vi "main 0.9.3.testing.vi"() -> ()   [LabVIEW 2015]
uses:
  subvi/PHOIBOS/DEFINITIONS/DEF_dev_state.ctl
  subvi/PHOIBOS/DEFINITIONS/DEF_dev_type.ctl
  <vilib>/Analysis/1siggen.llb/Ramp Pattern by Samples.vi
  <vilib>/Utility/file.llb/Write Delimited Spreadsheet (DBL).vi
  <vilib>/Utility/file.llb/Read Delimited Spreadsheet (string).vi
  <vilib>/DAQmx/create/channels.llb/DAQmx Create Channel (AI-Voltage-Basic).vi
  subvi/Newport ESP301/Newport ESP301.lvlib
  subvi/sp_manip.llb/sp_manip_lib.lvlib
  subvi/sp_manip.llb/tcp_gateway.lvlib
  <vilib>/Analysis/NI_AALBase.lvlib
panel:
  in  "Frame trigger \n(High Performance and QE only)":u16
  in  "Operating mode\nHP & QE / HS & DiCam Pro":u32
  out "Waveform Chart":dbl(graph)
  out "G2 X":cluster{dbl[], "Ramp Pattern":dbl[]}(graph)={array[344 elements], "Ramp Pattern"=[5593.0, 5541.0, 5578.0, 5573.0, 5542.0, 5582.0, 5523.0, 5570.0, 5578.0, 5560.0, 5581.0, 5542.0, 5577.0, 5517.0, 5599.0, 5558.0, 5549.0, 5571.0, 5527.0, 5574.0, 5565.0, 5561.0, 5570.0, 5531.0, 5576.0, 5531.0, 5576.0, 5554.0, 5523.0, 5573.0, 5536.0, 5555.0, 5539.0, 5549.0, 5543.0, 5541.0, 5581.0, 5523.0, 5548.0, 5528.0, 5558.0, 5565.0, 5537.0, 5556.0, 5521.0, 5538.0, 5549.0, 5532.0, 5562.0, 5512.0, 5555.0, 5549.0, 5536.0, 5542.0, 5511.0, 5567.0, 5526.0, 5549.0, 5545.0, 5543.0, 5562.0, 5518.0, 5561.0, 5490.0, 5542.0, 5522.0, 5529.0, 5542.0, 5521.0, 5556.0, 5511.0, 5541.0, 5534.0, 5512.0, 5569.0, 5525.0, 5547.0, 5507.0, 5533.0, 5533.0, 5501.0, 5555.0, 5497.0, 5517.0, 5526.0, 5519.0, 5565.0, 5503.0, 5548.0, 5496.0, 5544.0, 5523.0, 5534.0, 5533.0, 5501.0, 5529.0, 5494.0, 5523.0, 5526.0, 5519.0, 5539.0, 5493.0, 5508.0, 5532.0, 5504.0, 5546.0, 5540.0, 5550.0, 5488.0, 5556.0, 5535.0, 5510.0, 5535.0, 5515.0, 5543.0, 5475.0, 5538.0, 5528.0, 5504.0, 5523.0, 5502.0, 5535.0, 5473.0, 5503.0, 5501.0, 5531.0, 5525.0, 5490.0, 5524.0, 5484.0, 5520.0, 5506.0, 5492.0, 5516.0, 5477.0, 5511.0, 5487.0, 5509.0, 5496.0, 5467.0, 5538.0, 5494.0, 5512.0, 5497.0, 5498.0, 5526.0, 5482.0, 5506.0, 5466.0, 5522.0, 5489.0, 5512.0, 5518.0, 5475.0, 5547.0, 5480.0, 5569.0, 5504.0, 5485.0, 5528.0, 5506.0, 5529.0, 5468.0, 5524.0, 5507.0, 5518.0, 5511.0, 5471.0, 5525.0, 5480.0, 5482.0, 5510.0, 5506.0, 5522.0, 5475.0, 5540.0, 5477.0, 5511.0, 5514.0, 5500.0, 5497.0, 5484.0, 5536.0, 5476.0, 5485.0, 5527.0, 5509.0, 5529.0, 5495.0, 5504.0, 5496.0, 5519.0, 5512.0, 5469.0, 5506.0, 5465.0, 5502.0, 5481.0, 5508.0, 5519.0, 5499.0, 5515.0, 5476.0, 5496.0, 5502.0, 5499.0, 5494.0, 5477.0, 5541.0, 5477.0, 5512.0, 5497.0, 5472.0, 5511.0, 5471.0, 5503.0, 5507.0, 5504.0, 5477.0, 5479.0, 5508.0, 5481.0, 5522.0, 5517.0, 5516.0, 5505.0, 5502.0, 5491.0, 5481.0, 5512.0, 5484.0, 5500.0, 5478.0, 5493.0, 5529.0, 5492.0, 5518.0, 5471.0, 5518.0, 5490.0, 5513.0, 5497.0, 5488.0, 5517.0, 5477.0, 5524.0, 5464.0, 5495.0, 5514.0, 5495.0, 5522.0, 5477.0, 5490.0, 5535.0, 5489.0, 5491.0, 5491.0, 5515.0, 5473.0, 5504.0, 5505.0, 5515.0, 5510.0, 5473.0, 5521.0, 5475.0, 5537.0, 5499.0, 5505.0, 5509.0, 5460.0, 5509.0, 5473.0, 5489.0, 5500.0, 5464.0, 5522.0, 5471.0, 5528.0, 5475.0, 5502.0, 5494.0, 5511.0, 5516.0, 5486.0, 5528.0, 5471.0, 5492.0, 5477.0, 5491.0, 5531.0, 5486.0, 5549.0, 5498.0, 5524.0, 5482.0, 5495.0, 5505.0, 5476.0, 5512.0, 5444.0, 5512.0, 5498.0, 5471.0, 5489.0, 5462.0, 5502.0, 5459.0, 5503.0, 5489.0, 5493.0, 5498.0, 5461.0, 5505.0, 5495.0, 5503.0, 5459.0, 5501.0, 5515.0, 5459.0, 5510.0, 5469.0, 5504.0, 5499.0, 5505.0, 5524.0, 5477.0, 5527.0, 5477.0, 5475.0, 5495.0, 5482.0, 5514.0, 5481.0, 5499.0, 5481.0, 5482.0, 5498.0, 5460.0, 5469.0, 5471.0, 5519.0, 5495.0, 5485.0]}
  in  "reset every n pics":bool
  in  "pics2avg":i32=50
  in  "abort acq.":bool
  out "G2 Y":cluster{dbl[], "Ramp Pattern":dbl[]}(graph)={[5738.0, 5692.0, 5562.0, 5630.0, 5633.0, 5616.0, 5523.0, 5622.0, 5406.0, 5598.0, 5416.0, 5403.0, 5579.0, 5325.0, 5504.0, 5402.0, 5538.0, 5568.0, 5460.0, 5494.0, 5367.0, 5597.0, 5434.0, 5448.0, 5339.0, 5434.0, 5460.0, 5482.0, 5646.0, 5720.0, 5704.0, 5628.0, 5672.0, 5511.0, 5420.0, 5539.0, 5543.0, 5421.0, 5486.0, 5508.0, 5537.0, 5586.0, 5460.0, 5547.0, 5433.0, 5488.0, 5552.0, 5538.0, 5528.0, 5482.0, 5406.0, 5458.0, 5644.0, 5485.0, 5443.0, 5485.0, 5385.0, 5413.0, 5472.0, 5571.0, 5640.0, 5602.0, 5462.0, 5477.0, 5408.0, 5396.0, 5445.0, 5638.0, 5383.0, 5571.0, 5372.0, 5519.0, 5426.0, 5462.0, 5481.0, 5626.0, 5326.0, 5458.0, 5471.0, 5366.0, 5394.0, 5363.0, 5551.0, 5596.0, 5452.0, 5470.0, 5600.0, 5533.0, 5573.0, 5544.0, 5671.0, 5595.0, 5423.0, 5550.0, 5557.0, 5416.0, 5404.0, 5478.0, 5448.0, 5512.0, 5505.0, 5575.0, 5434.0, 5436.0, 5600.0, 5487.0, 5607.0, 5463.0, 5606.0, 5540.0, 5521.0, 5581.0, 5472.0, 5555.0, 5576.0, 5612.0, 5529.0, 5473.0, 5454.0, 5455.0, 5500.0, 5650.0, 5451.0, 5445.0, 5423.0, 5376.0, 5389.0, 5491.0, 5536.0, 5525.0, 5440.0, 5707.0, 5414.0, 5532.0, 5400.0, 5668.0, 5706.0, 5515.0, 5431.0, 5400.0, 5439.0, 5471.0, 5627.0, 5691.0, 5569.0, 5718.0, 5614.0, 5523.0, 5436.0, 5432.0, 5419.0, 5516.0, 5469.0, 5467.0, 5530.0, 5598.0, 5501.0, 5476.0, 5457.0, 5460.0, 5606.0, 5456.0, 5429.0, 5586.0, 5504.0, 5546.0, 5516.0, 5466.0, 5650.0, 5593.0, 5605.0, 5515.0, 5414.0, 5623.0, 5581.0, 5651.0, 5574.0, 5519.0, 5672.0, 5621.0, 5496.0, 5382.0, 5496.0, 5620.0, 5542.0, 5422.0, 5492.0, 5515.0, 5549.0, 5402.0, 5472.0, 5547.0, 5515.0, 5641.0, 5451.0, 5667.0, 5622.0, 5511.0, 5506.0, 5608.0, 5647.0, 5584.0, 5714.0, 5490.0, 5534.0, 5463.0, 5566.0, 5573.0, 5570.0, 5582.0, 5613.0, 5504.0, 5550.0, 5594.0, 5576.0, 5677.0, 5675.0, 5681.0, 5681.0, 5434.0, 5434.0, 5405.0, 5473.0, 5522.0, 5427.0, 5533.0, 5582.0, 5427.0, 5529.0, 5548.0, 5341.0, 5521.0, 5539.0, 5435.0, 5457.0, 5511.0, 5406.0, 5412.0, 5620.0, 5609.0, 5609.0, 5469.0, 5577.0, 5661.0, 5673.0, 5518.0, 5463.0, 5562.0, 5723.0, 5719.0, 5487.0, 5485.0, 5683.0, 5501.0, 5604.0, 5328.0], "Ramp Pattern"=[0.0, 1.003921568627451, 2.007843137254902, 3.011764705882353, 4.015686274509804, 5.019607843137255, 6.023529411764706, 7.027450980392157, 8.031372549019608, 9.035294117647059, 10.03921568627451, 11.04313725490196, 12.047058823529412, 13.050980392156863, 14.054901960784314, 15.058823529411764, 16.062745098039215, 17.066666666666666, 18.070588235294117, 19.07450980392157, 20.07843137254902, 21.08235294117647, 22.08627450980392, 23.090196078431372, 24.094117647058823, 25.098039215686274, 26.101960784313725, 27.105882352941176, 28.109803921568627, 29.113725490196078, 30.11764705882353, 31.12156862745098, 32.12549019607843, 33.129411764705885, 34.13333333333333, 35.13725490196079, 36.141176470588235, 37.14509803921569, 38.14901960784314, 39.15294117647059, 40.15686274509804, 41.16078431372549, 42.16470588235294, 43.168627450980395, 44.17254901960784, 45.1764705882353, 46.180392156862744, 47.1843137254902, 48.188235294117646, 49.1921568627451, 50.19607843137255, 51.2, 52.20392156862745, 53.207843137254905, 54.21176470588235, 55.21568627450981, 56.219607843137254, 57.22352941176471, 58.227450980392156, 59.23137254901961, 60.23529411764706, 61.23921568627451, 62.24313725490196, 63.247058823529414, 64.25098039215686, 65.25490196078431, 66.25882352941177, 67.26274509803922, 68.26666666666667, 69.27058823529411, 70.27450980392157, 71.27843137254902, 72.28235294117647, 73.28627450980392, 74.29019607843138, 75.29411764705883, 76.29803921568627, 77.30196078431372, 78.30588235294118, 79.30980392156863, 80.31372549019608, 81.31764705882352, 82.32156862745099, 83.32549019607843, 84.32941176470588, 85.33333333333333, 86.33725490196079, 87.34117647058824, 88.34509803921569, 89.34901960784313, 90.3529411764706, 91.35686274509804, 92.36078431372549, 93.36470588235294, 94.3686274509804, 95.37254901960785, 96.37647058823529, 97.38039215686274, 98.3843137254902, 99.38823529411765, 100.3921568627451, 101.39607843137254, 102.4, 103.40392156862745, 104.4078431372549, 105.41176470588235, 106.41568627450981, 107.41960784313726, 108.4235294117647, 109.42745098039215, 110.43137254901961, 111.43529411764706, 112.43921568627451, 113.44313725490196, 114.44705882352942, 115.45098039215686, 116.45490196078431, 117.45882352941176, 118.46274509803922, 119.46666666666667, 120.47058823529412, 121.47450980392156, 122.47843137254903, 123.48235294117647, 124.48627450980392, 125.49019607843137, 126.49411764705883, 127.49803921568628, 128.50196078431372, 129.50588235294117, 130.50980392156862, 131.51372549019607, 132.51764705882354, 133.521568627451, 134.52549019607844, 135.52941176470588, 136.53333333333333, 137.53725490196078, 138.54117647058823, 139.54509803921567, 140.54901960784315, 141.5529411764706, 142.55686274509804, 143.5607843137255, 144.56470588235294, 145.5686274509804, 146.57254901960783, 147.57647058823528, 148.58039215686276, 149.5843137254902, 150.58823529411765, 151.5921568627451, 152.59607843137255, 153.6, 154.60392156862744, 155.6078431372549, 156.61176470588236, 157.6156862745098, 158.61960784313726, 159.6235294117647, 160.62745098039215, 161.6313725490196, 162.63529411764705, 163.6392156862745, 164.64313725490197, 165.64705882352942, 166.65098039215687, 167.65490196078431, 168.65882352941176, 169.6627450980392, 170.66666666666666, 171.6705882352941, 172.67450980392158, 173.67843137254903, 174.68235294117648, 175.68627450980392, 176.69019607843137, 177.69411764705882, 178.69803921568626, 179.7019607843137, 180.7058823529412, 181.70980392156864, 182.71372549019608, 183.71764705882353, 184.72156862745098, 185.72549019607843, 186.72941176470587, 187.73333333333332, 188.7372549019608, 189.74117647058824, 190.7450980392157, 191.74901960784314, 192.75294117647059, 193.75686274509803, 194.76078431372548, 195.76470588235293, 196.7686274509804, 197.77254901960785, 198.7764705882353, 199.78039215686275, 200.7843137254902, 201.78823529411764, 202.7921568627451, 203.79607843137254, 204.8, 205.80392156862746, 206.8078431372549, 207.81176470588235, 208.8156862745098, 209.81960784313725, 210.8235294117647, 211.82745098039214, 212.83137254901962, 213.83529411764707, 214.8392156862745, 215.84313725490196, 216.8470588235294, 217.85098039215686, 218.8549019607843, 219.85882352941175, 220.86274509803923, 221.86666666666667, 222.87058823529412, 223.87450980392157, 224.87843137254902, 225.88235294117646, 226.8862745098039, 227.89019607843136, 228.89411764705883, 229.89803921568628, 230.90196078431373, 231.90588235294118, 232.90980392156862, 233.91372549019607, 234.91764705882352, 235.92156862745097, 236.92549019607844, 237.9294117647059, 238.93333333333334, 239.93725490196078, 240.94117647058823, 241.94509803921568, 242.94901960784313, 243.95294117647057, 244.95686274509805, 245.9607843137255, 246.96470588235294, 247.9686274509804, 248.97254901960784, 249.9764705882353, 250.98039215686273, 251.98431372549018, 252.98823529411766, 253.9921568627451, 254.99607843137255, 256.0]}
  out "ETA":timestamp=timestamp(3543843884.995538 s since 1904-01-01) format="%<%H:%M:%S>T"
  out "acq. imgs":i32=30
  out "snap_prog":dbl(slide)=1.0 scale=0.0..1.0
  in  "BasePath":path=path "Z:/PESdata"
  in  "cam_liveavg":bool caption="live average"
  out "cam_fps":dbl=20.079713544692744 caption="FPS" format="%.1g"
  out "sideimg":dbl[][](graph)
  in  "RunNumber":u16=77
  out "sum":dbl=4126991.0 format="%#.2g"
  out "max":dbl=54.0
  out "mainimg":dbl[][](graph)
  out "ESP_con?":bool=TRUE caption="ESP301"
  out "phoib_con?":bool caption="PHOIBOS"
  out "manip_con?":bool caption="manipulator"
  out "cam_con?":bool caption="camera"
  in  "main_close":bool
  in  "Tab Control":T1(tab)
  in  "manip_deltas":dbl[](array[numeric])=[0.0, 0.0, 0.0, 0.0, 10.0, 0.0] caption="delta" format="%#.5g"
  in  "aq.mode":enum32{"Radio Selection 1", "Radio Selection 2"}(radio)=enum."Radio Selection 2"
  in  "dark avg":i32=100
  in  "averages":i32=30 caption="N"
  in  "ESP_delta":dbl caption="relative [mm]"
  in  "ESP_-":bool
  in  "ESP_+":bool
  in  "ESP_go":bool
  in  "ESP_dest_t":dbl=250.17307139859977 caption="[fs]"
  in  "ESP_dest":dbl=31.304 caption="[mm]"
  in  "ESP_set_t0":bool
  in  "phoib_I_6s":dbl=3200.0
  in  "phoib_I_5s":dbl=1650.0
  in  "phoib_I_4s":dbl=4.558
  in  "phoib_I_3s":dbl=-7.0
  in  "phoib_I_2s":dbl=20.0
  in  "phoib_I_1s":dbl=22.0
  in  "phoib_standby":bool
  in  "phoib_set":bool
  out "phoib_I_6":dbl caption="Screen Voltage"
  out "phoib_I_5":dbl caption="Detctor Voltage"
  out "phoib_I_4":dbl caption="Work Function"
  out "phoib_I_3":dbl caption="Coil Current"
  out "phoib_I_2":dbl caption="Pass Energy"
  out "phoib_I_1":dbl caption="Kinetic Energy"
  out "Saved Positions":string[][](table)=[["ertwertwert", "-2.299945", "-2.030214", "38.900024", "50.000762", "0.000887", "-97.998082"], ["uztgugt", "-14.999451", "-13.638894", "442.380066", "13.998380", "-1.893758", "-76.305838"], ["asdf", "-14.999451", "-13.638894", "442.380066", "13.998380", "-1.893758", "-76.305838"], ["test3", "-14.999451", "-13.638894", "441.380066", "13.998380", "-1.893758", "-76.305838"]]
  in  "Save Pos":bool
  in  "Load":bool
  in  "Delete":bool
  in  "ManipRel +":bool
  in  "ManipRel -":bool
  in  "Move Abs":bool
  in  "stop manip":bool
  in  "dest":dbl[](array[numeric])=[-2.6172862113166087, -0.009888298846365134, 68.5008544921875, -46.36280498847848, 1.1073518432055398, -218.56360350415366] caption="destination" format="%#.5g"
  out "axis":string[](array[string])=["x", "y", "z", "polar", "tilt", "azimut"]
  out "pos":dbl[](array[numeric])=[-2.6172862113166087, -0.009888298846365134, 68.5008544921875, -46.363686276590336, 11.108982061941884, -218.56360350415366] caption="position" format="%.5f"
  in  "Mode":T2(ring)=enum."WideAngleMode"
  in  "VoltageRange":enum16{"3.5kV", "1.5kV", "400V", "100V", "10V"}(ring)=enum."400V"
  out "ESP_pos":dbl=31.4539 caption="Position"
  out "ESP_delay":dbl=1000.0251574040756 caption="Delay"
  out "ESP_t0":dbl=31.304 caption="Time Zero @"
  out "phoib_I_7":dbl caption="Conversion Voltage"
  in  "phoib_I_7s":dbl=-16.0
  in  "phoib_I_8s":dbl=0.0039
  in  "phoib_I_9s":dbl=0.0039
  out "phoib_I_8":dbl caption="FD1"
  out "phoib_I_9":dbl caption="FD2"
  in  "gain":bool
  in  "exposure [ms]":u32=1
  in  "binning":u16(ring)=2 items=["X 1", "X 2", "X 4", "X 8"]
  in  "cam_dark?":bool caption="subtract dark?"
  in  "cam_dark":bool
  in  "cam_saveimg":bool
  in  "e-size":u8
  in  "lower threshold":i32=-100
  in  "count?":bool
  in  "ROI Left":i32=1
  in  "ROI Right":i32=43
  in  "ROI Top":i32=1
  in  "ROI Bottom":i32=33
  out "moving?":bool[](array[boolean])
  in  "delscan_abort 2":bool
  in  "delscan_go 2":bool
  in  "delscan_finishIteration 2":bool
  out "del_ETA":timestamp=timestamp(3543843871.185777 s since 1904-01-01) format="%<%H:%M:%S>T"
  out "time / step":dbl=2.792118032773336
  out "duration [HH:MM:SS]":dbl=55.62603882380894 format="%<%H:%M:%S>t"
  out "disk [MB]":dbl=11.613000000000001
  out "RAM [MB]":dbl=2.765
  out "total steps":dbl=20.0
  out "delaypoints":dbl=5.0
  in  "generate delay table":bool
  in  "load delay table":bool
  in  "delay table [fs]":string[][](table)=[["-1000.000000"], ["-500.000000"], ["0.000000"], ["500.000000"], ["1000.000000"]]
  in  "delscan_iters":u32=4 caption="iterations"
  out "scangraph":cluster{"delaypoints":dbl[], dbl[]}(graph)={"delaypoints"=[-1000.0, -500.0, 0.0, 500.0, 1000.0], [56872639.0, 56944859.59999999, 56835838.7999999, 56879783.599999934, 56864774.39999998]}
  in  "delscan_abort":bool
  out "delscan_progress":u32(slide)=5 scale=0.0..5.0
  in  "delscan_go":bool
  out "delscan_pos":dbl=31.453896228999998 caption="stage pos [mm]"
  in  "delscan_end":dbl=1000.0 caption="end [fs]"
  in  "delscan_stepsize":dbl=500.0 caption="stepsize [fs]"
  in  "delscan_start":dbl=-1000.0 caption="start [fs]"
  out "iteration":i32=5
  in  "delscan_finishIteration":bool
  in  "manip_scan_steps":u32=3
  in  "Optimize":bool
  in  "manip_scan_delta":dbl[](array[numeric])=[0.0, 0.0, 0.0, 0.0, 1.0, 0.0] caption="delta" format="%#.5g"
  out "delscan_progress 2":u32(slide)=2 scale=0.0..3.0
  in  "abort":bool
  in  "dev_bench":bool
  out "x/y":dbl
  out "1/x":dbl
  in  "stop":bool
  out "voltage out":dbl
  out "sideimg 2":i32[][](graph)
  in  "manip_init":bool
  in  "manip_release":bool
  in  "phoib_init":bool
  in  "phoib_release":bool
  in  "ESP_init":bool
  in  "ESP_release":bool
  in  "ESP301 VISA":refnum<visa-resource-name>="COM8"
  in  "board number":i32
  in  "cam_init":bool
  in  "cam_release":bool
  out "cam_error":errorcluster
  out "phoib_error":errorcluster
  out "state":T3 items=["Off"=-1, "Standby"=0, "On"=1]
  in  "ESP Axis":i32=1 min=1 max=3
  out "error out":errorcluster
  out "error out 2":errorcluster={"status"=TRUE, "code"=1, "source"="TCP Write in sp_manip_lib.lvlib:sp_manip_disconnect.vi->main 0.9.1.vi"}
  # "0 = sequential\n1 = simultaneous"
  # "0 = internal\n1 = external rising\n2 = external falling"
  # "camera"
  # "analyzer"
  # "manipulator"
  # "aquisition"
  # "delay stage"
  # "Position"
  # "Destination"
  # "X\nY\nZ\npolar\ntilt\nazimut"
  # "camera"
  # "phoibos"
  # "ESP301"
  # "manipulator"
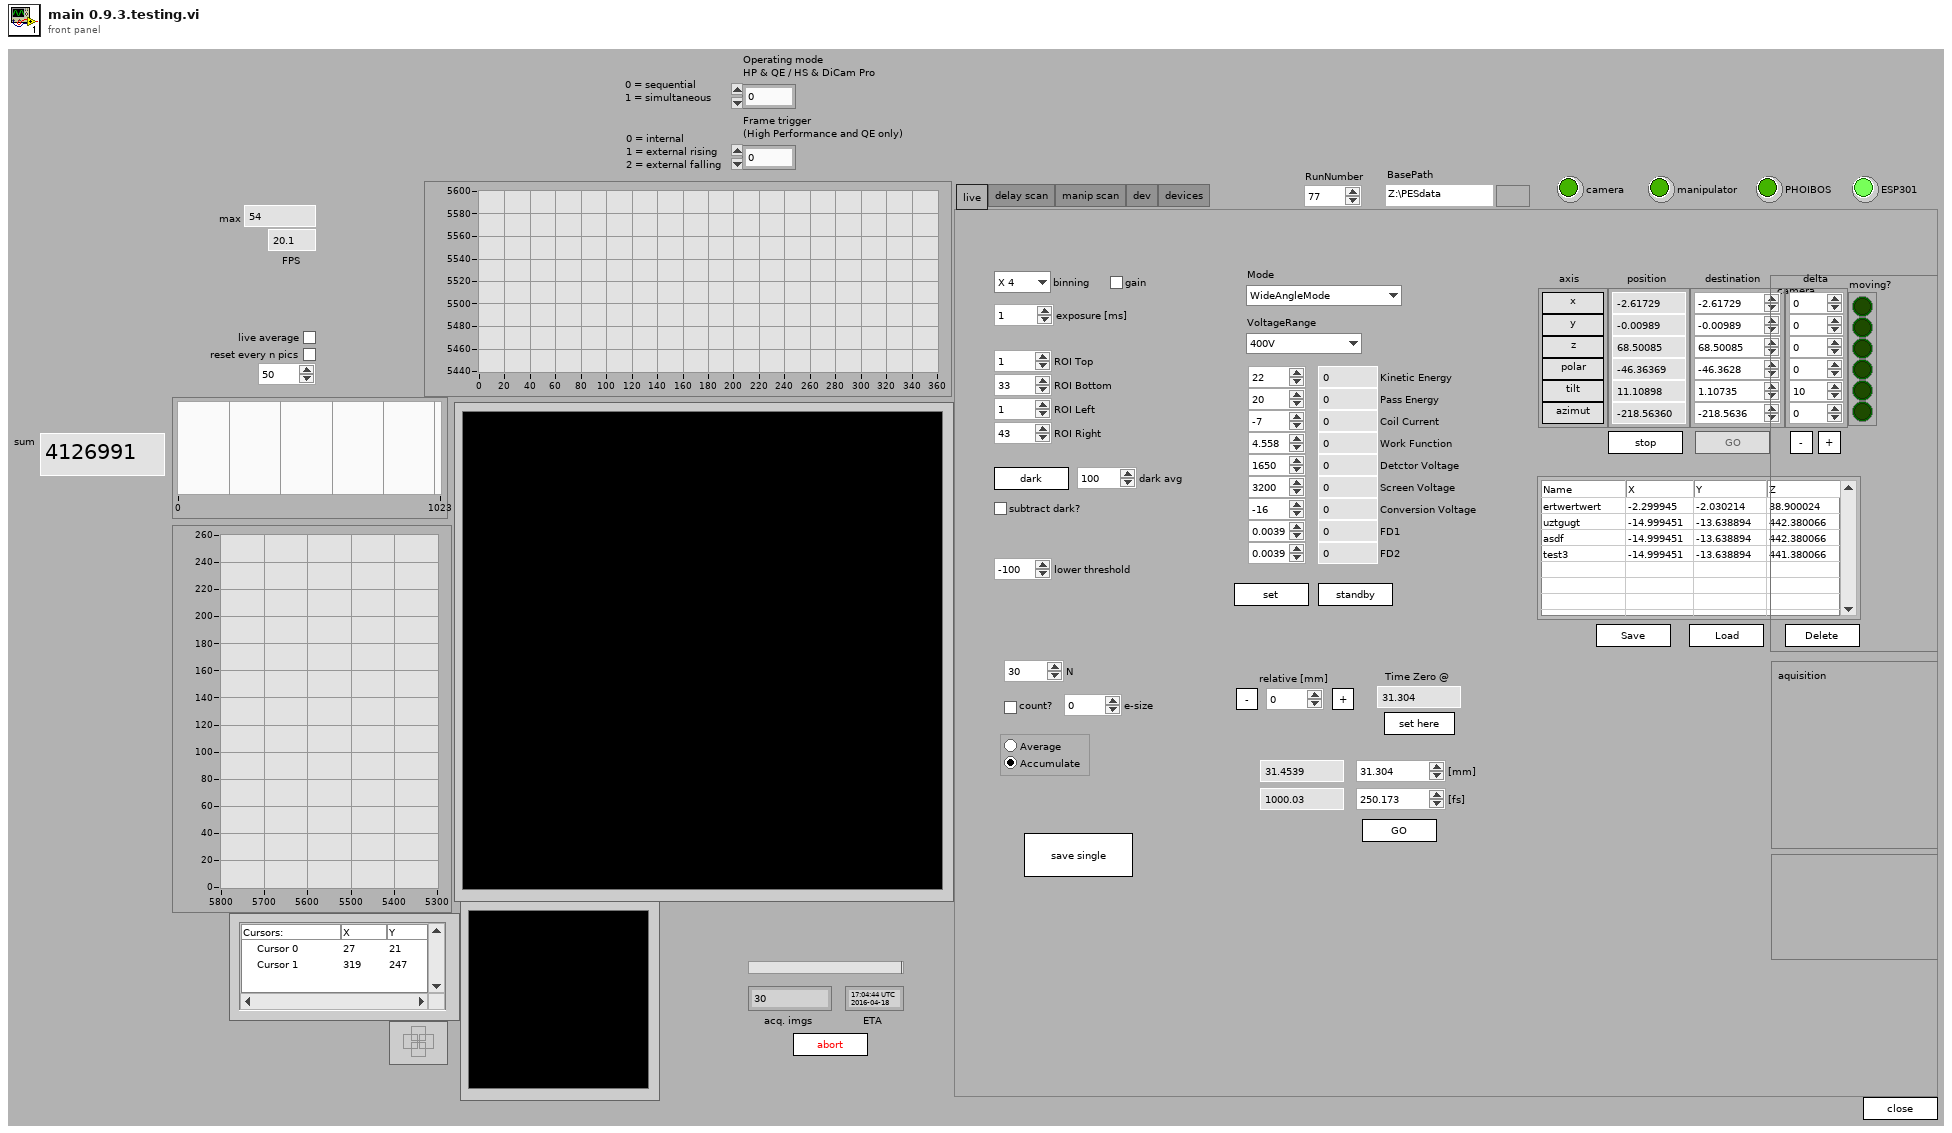
[diagram p1: front panel]
types:
  T1 = enum32{"live", "delay scan", "manip scan", "dev", "devices"}
  T2 = enum16{"HighMagnification", "MediumMagnification", "LowMagnification", "HighAngularDispersion", "MediumAngularDispersion", "LowAngularDispersion", "WideAngleMode", "LargeArea", "MediumArea", "SmallArea", "HighMagnification2", "SmallArea2", "ImagingMode"}
  T3 = typedef "DEF_dev_state.ctl" = i32
  T4 = typedef "LVCursorListTypeDef.ctl" = cluster{"Name":string, "Color":u32, "Style":u8, "Point Style":u8, "Name Visible":bool, "Allow Drag":bool, "Cursor Mode":u32, "Plot":i32, "Index":i32, "Position":cluster{"X":dbl, "Y":dbl}, "X Scale":u32, "Y Scale":u32, "Watch Plots":i32[], "Watch All Plots":bool, "Plot Area":i32, "Label Offset":cluster{"X":dbl, "Y":dbl}}[]
  T5 = cluster{"delay pointss [fs]":dbl[], "Intensity Chart":dbl[]}
  T6 = cluster{"Camera type":u32, "Operating mode\nHP & QE / HS & DiCam Pro ":u32, "Frame trigger \n(High Performance and QE only)":u16, "Sequence trigger":u16, "Low Light\n(QE only)":bool, "Gain":bool, "Horzontal\nbinning":u16, "Vertical\nbinning ":u16, "ROI Left":i32, "ROI Right":i32, "ROI Top":i32, "ROI Bottom":i32}
  T7 = cluster{"Name":string, "Color":u32, "Style":u8, "Point Style":u8, "Name Visible":bool, "Allow Drag":bool, "Cursor Mode":u32, "Plot":i32, "Index":i32, "Position":cluster{"X":dbl, "Y":dbl}, "X Scale":u32, "Y Scale":u32, "Watch Plots":i32[], "Watch All Plots":bool, "Plot Area":i32, "Label Offset":cluster{"X":dbl, "Y":dbl}}
  T8 = cluster{"Axis_Name":string, "Axis_Type":string, "Axis_Position":dbl, "continous":bool, "moving":bool}[]
  T9 = typedef "DEF_dev_type.ctl" = enum32{"devA (analyzer)", "devD (detector)"}
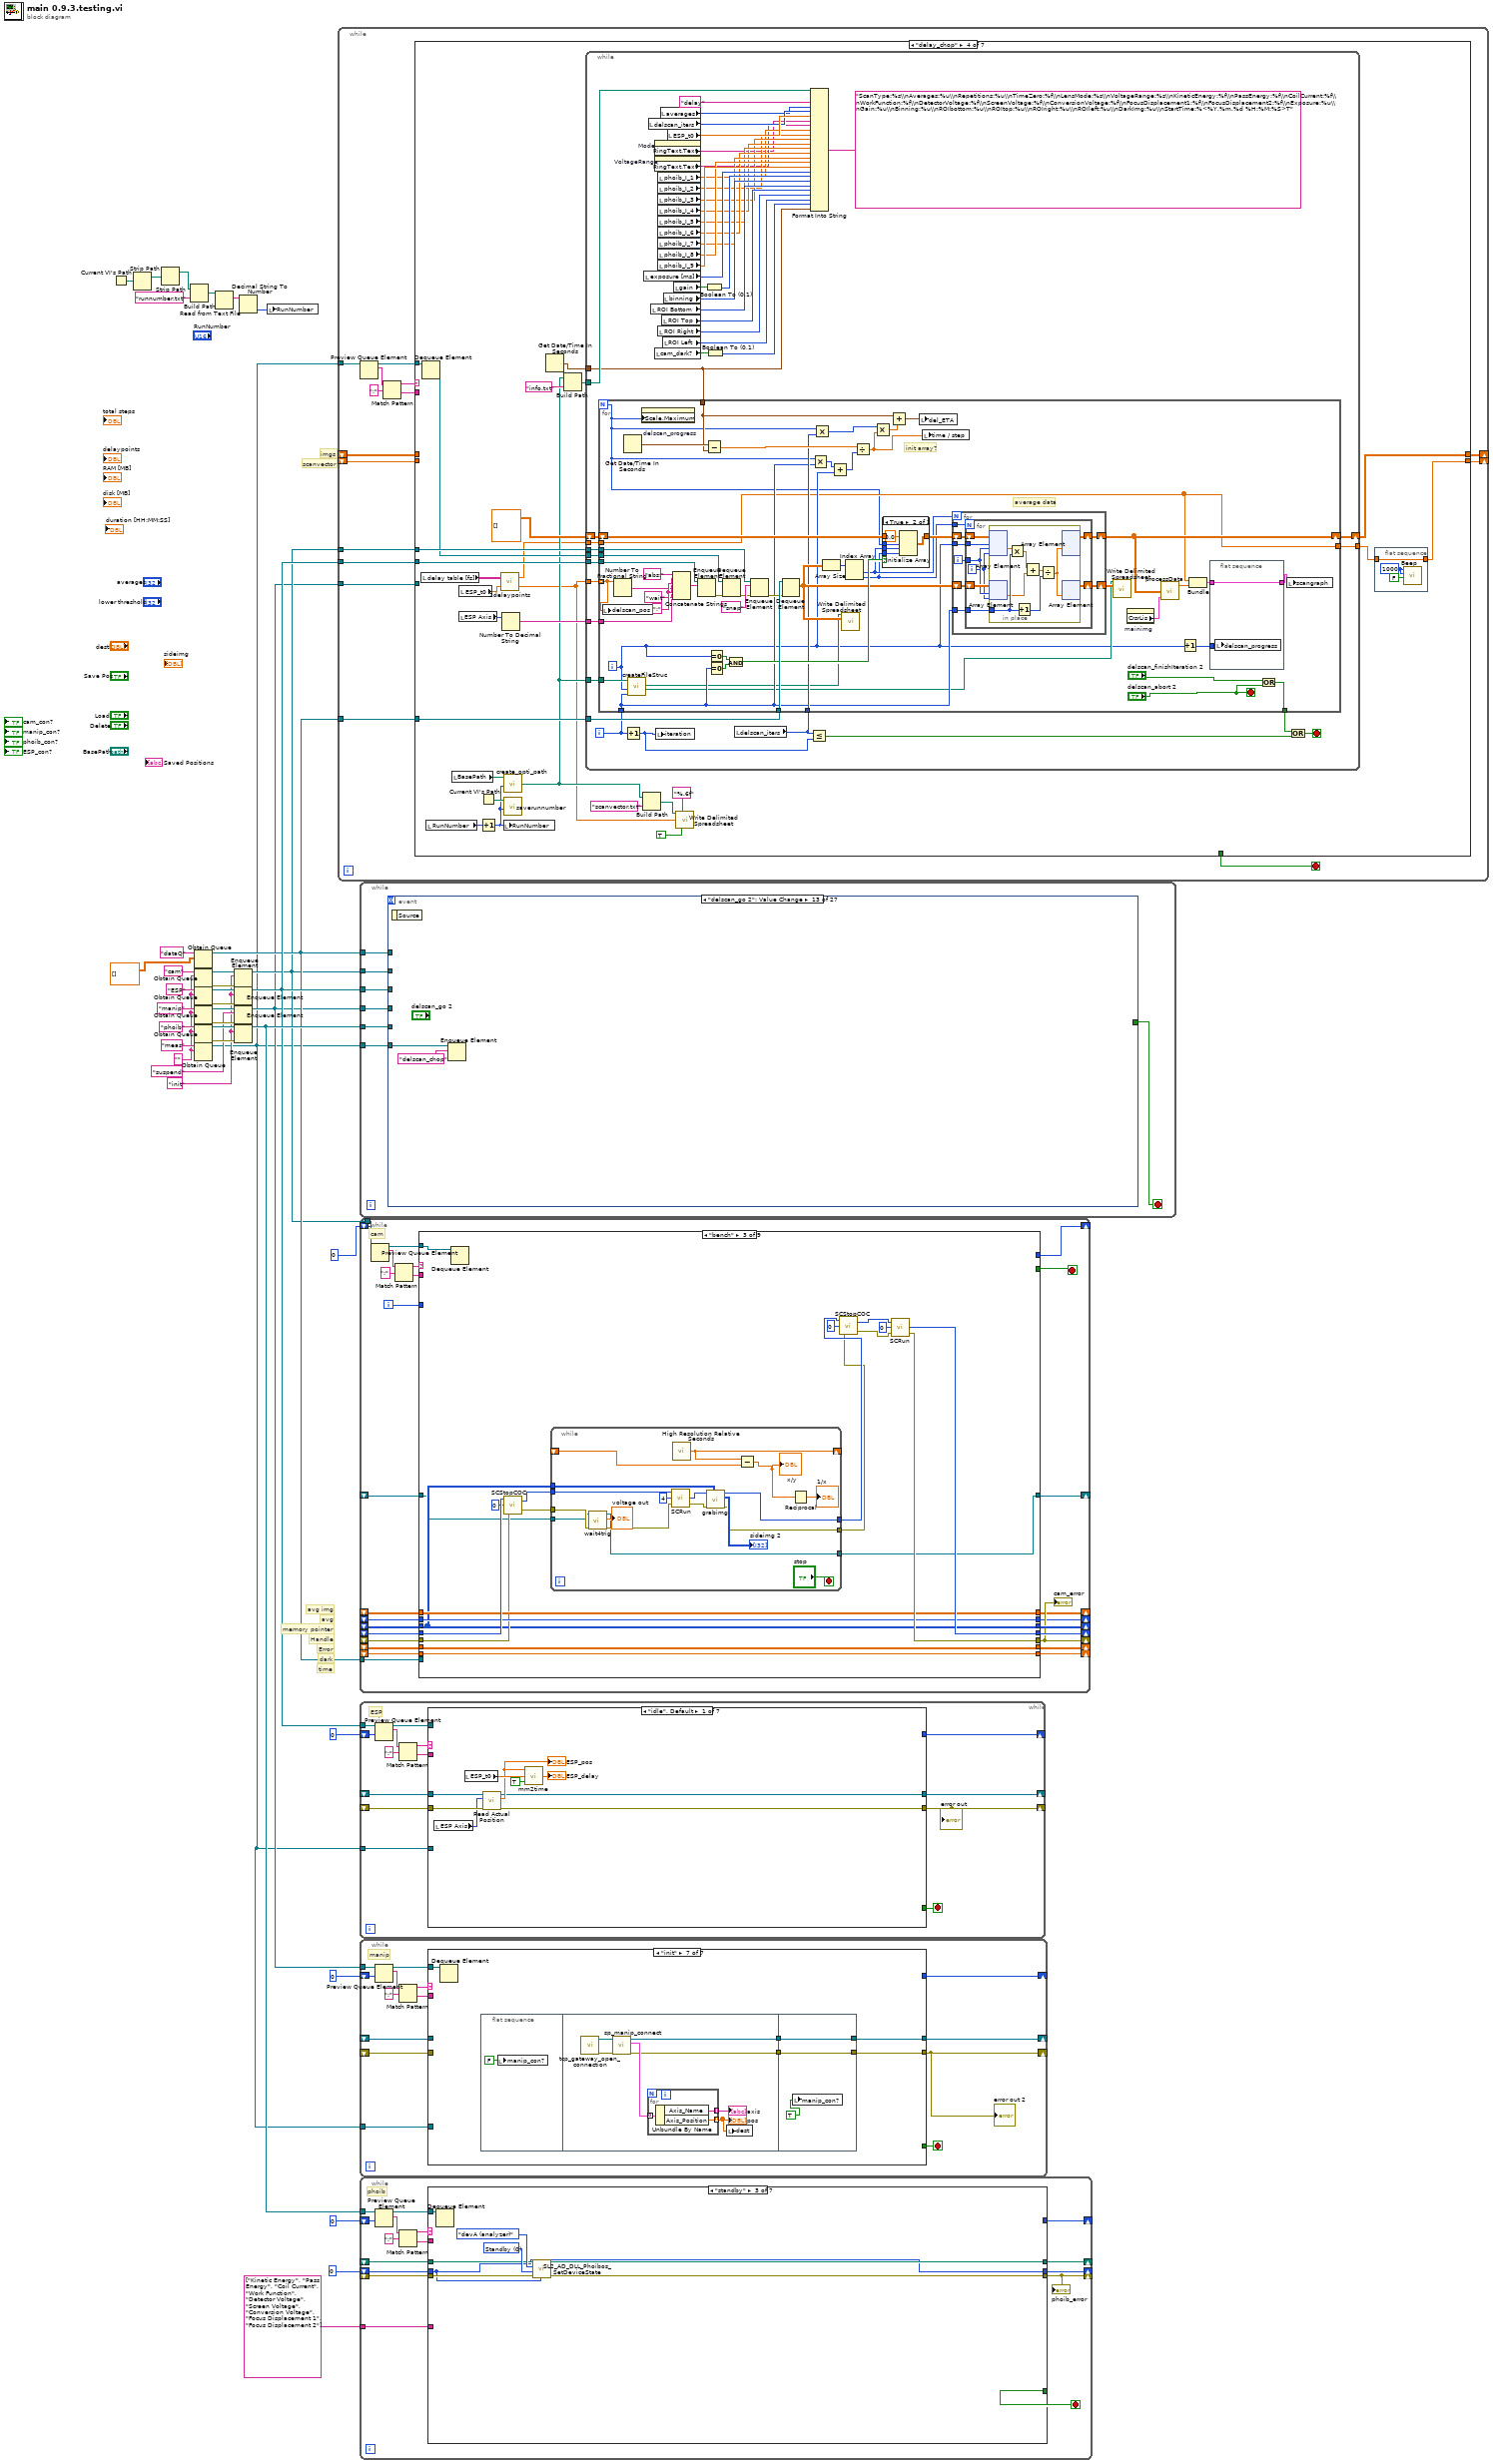
[diagram p0: block diagram]
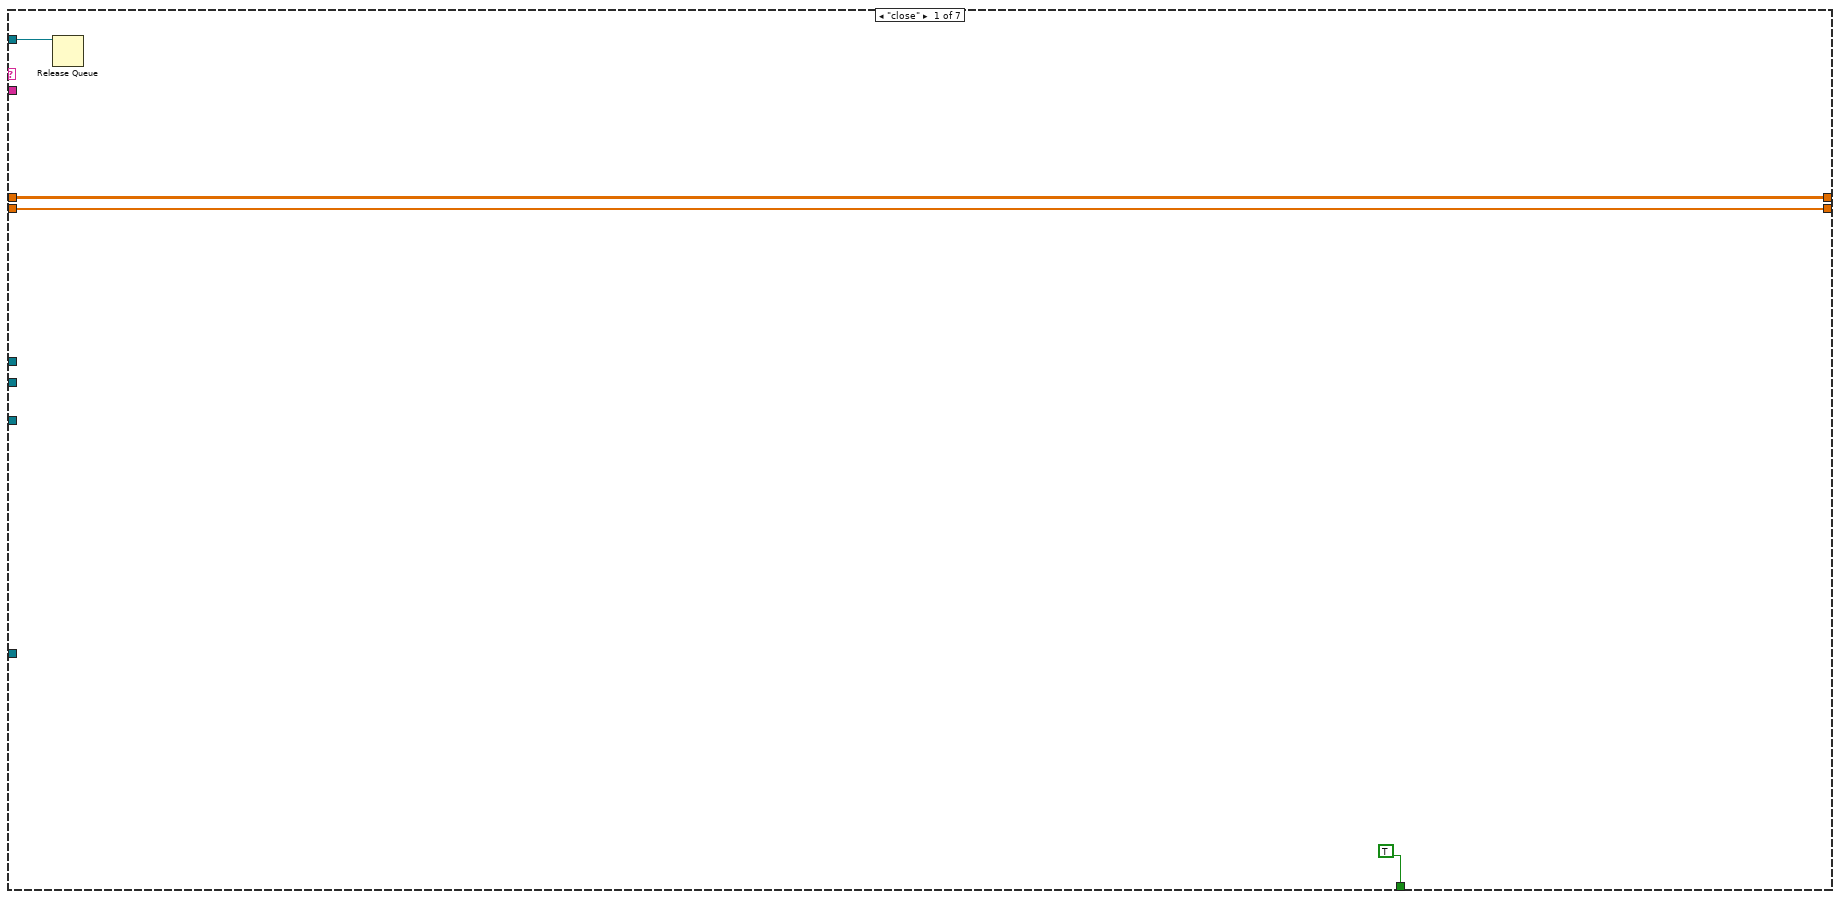
[diagram p2: hidden frame]
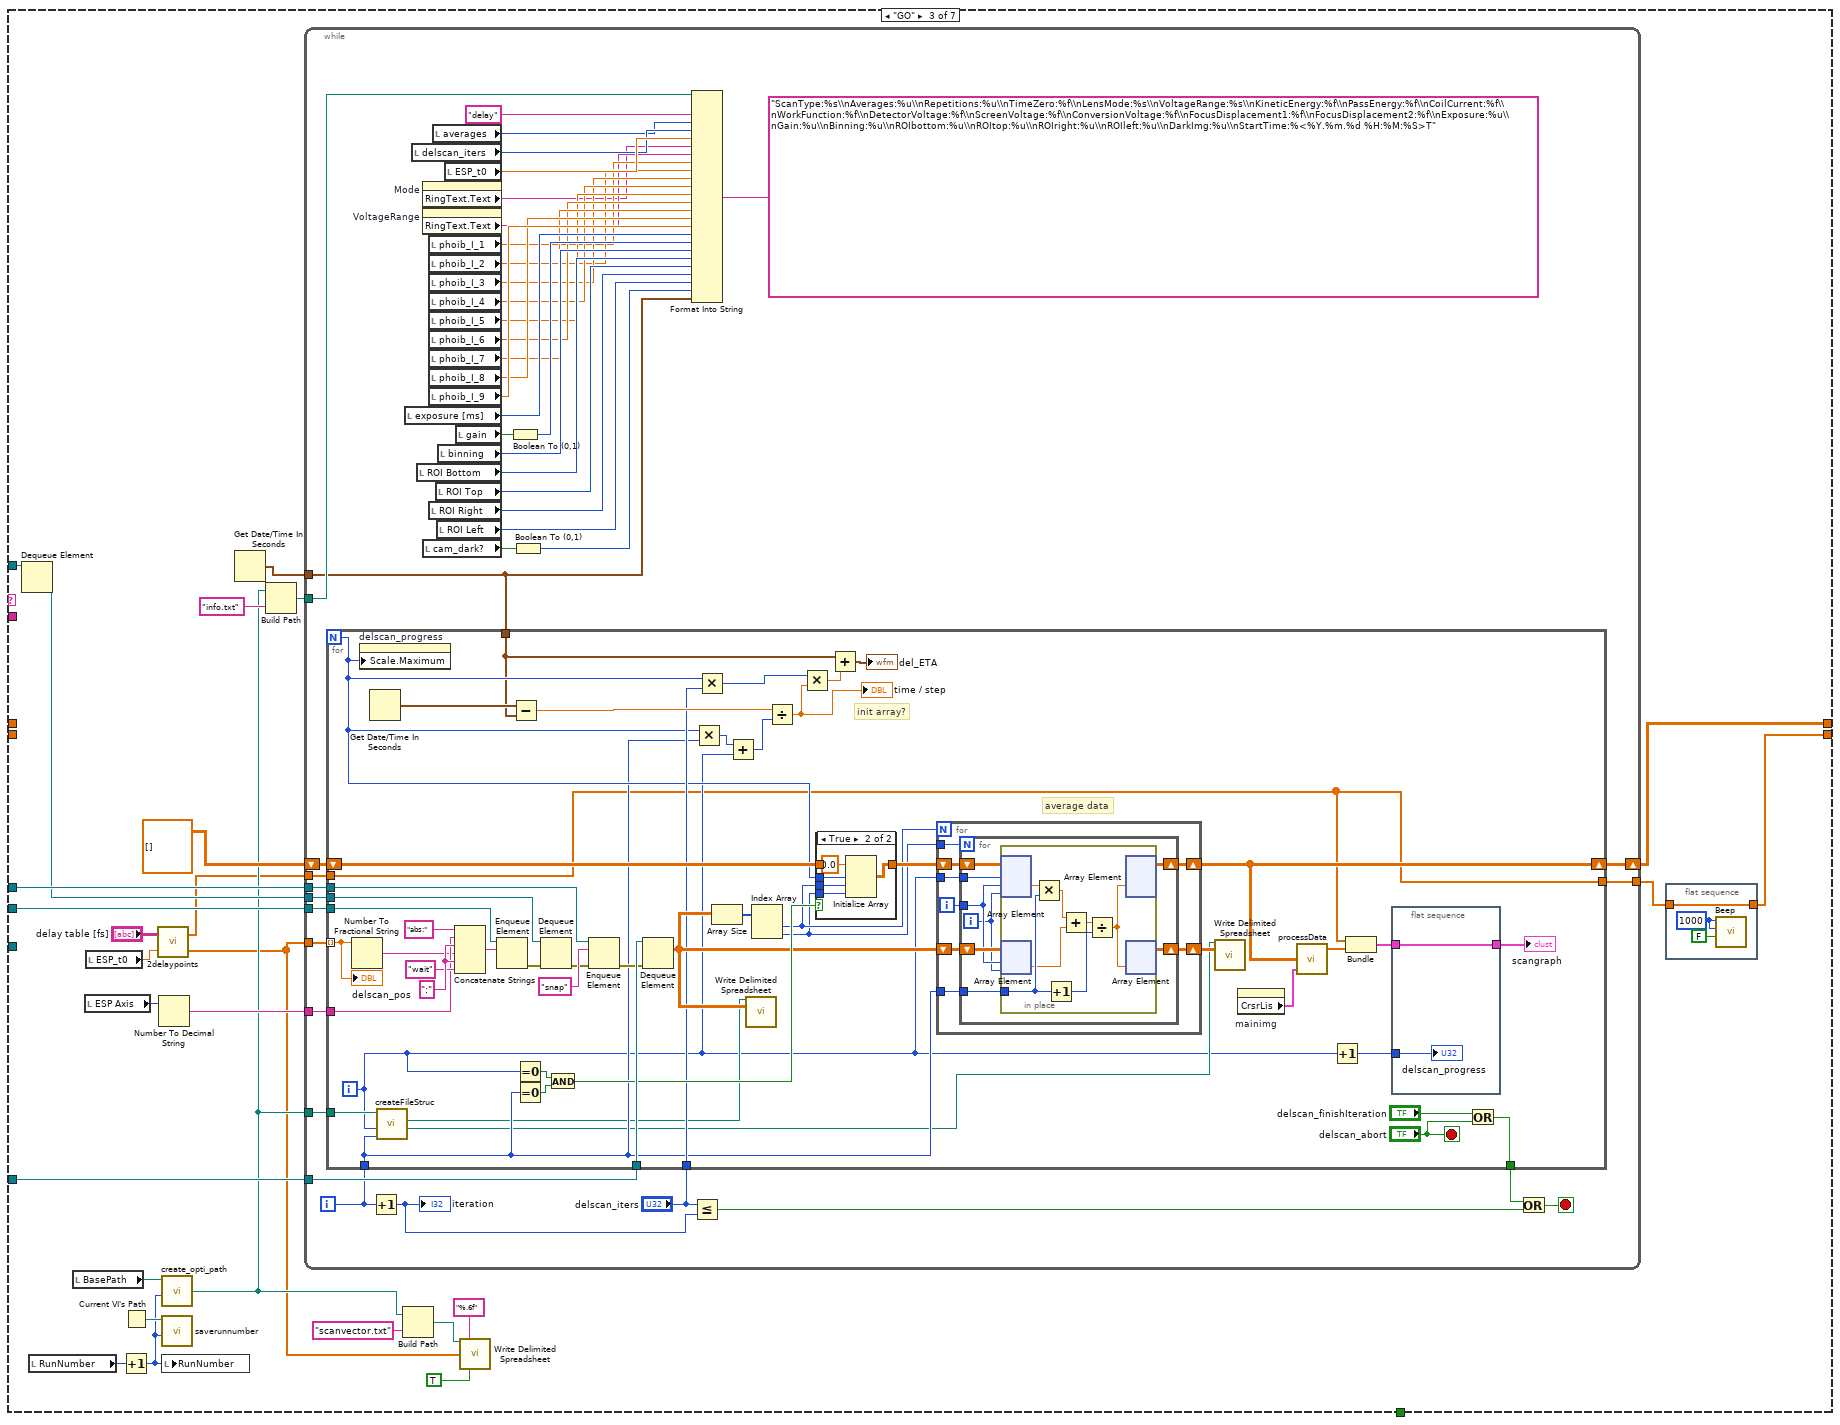
[diagram p4: hidden frame]
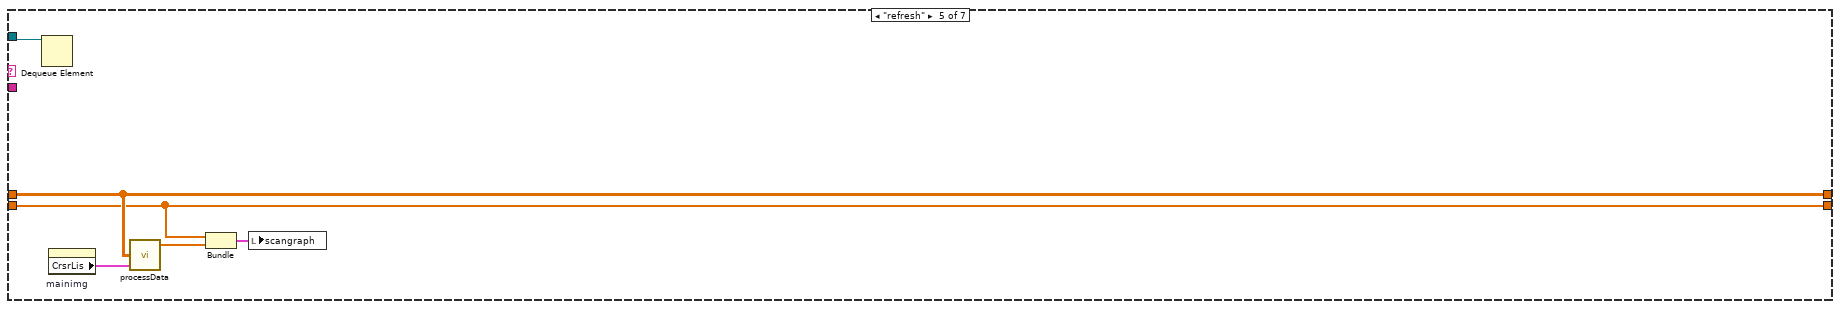
[diagram p7: hidden frame]
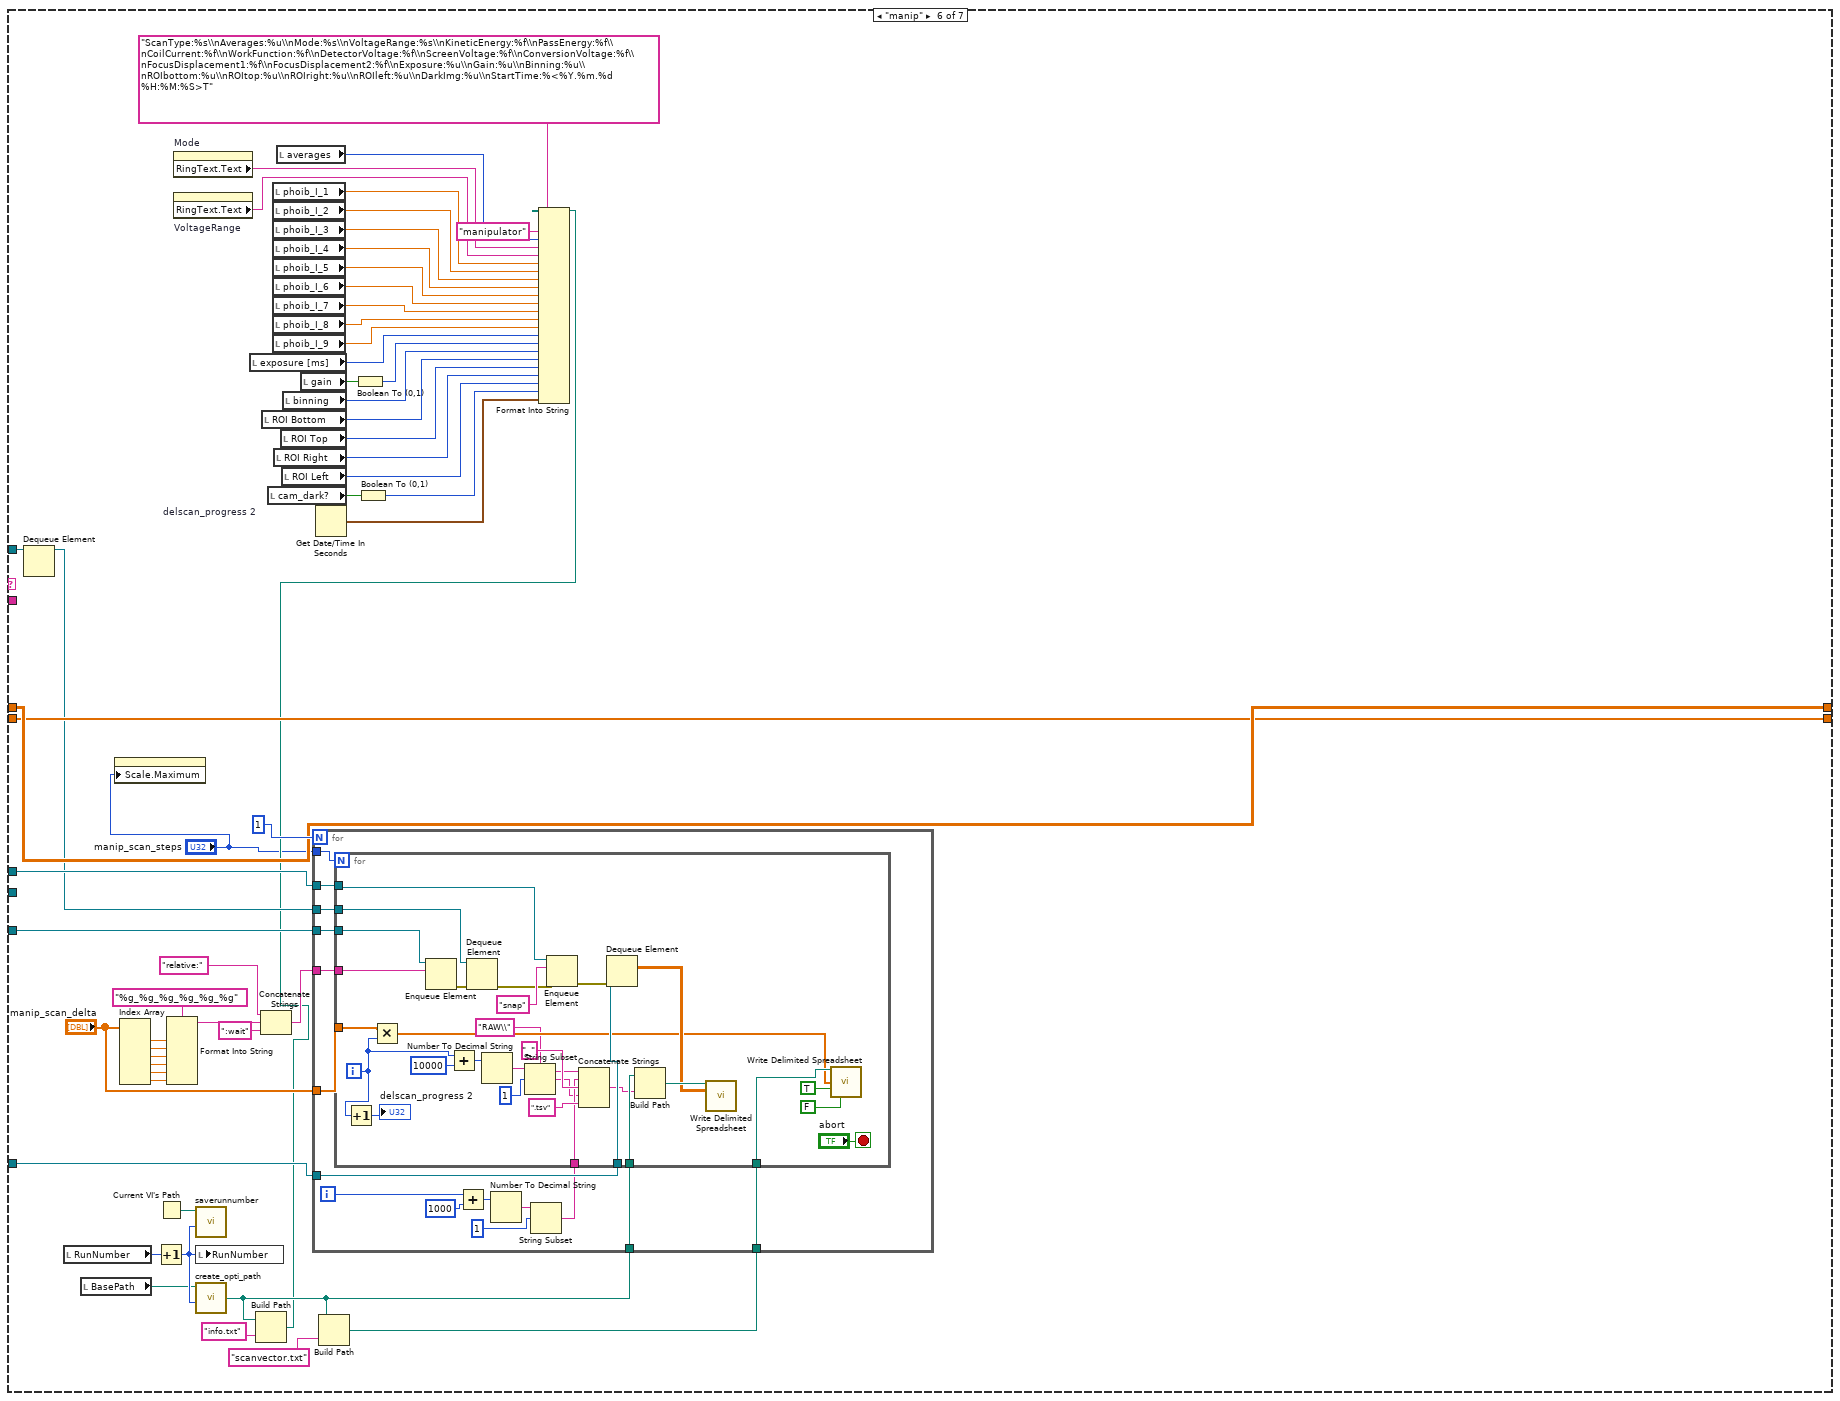
[diagram p8: hidden frame]
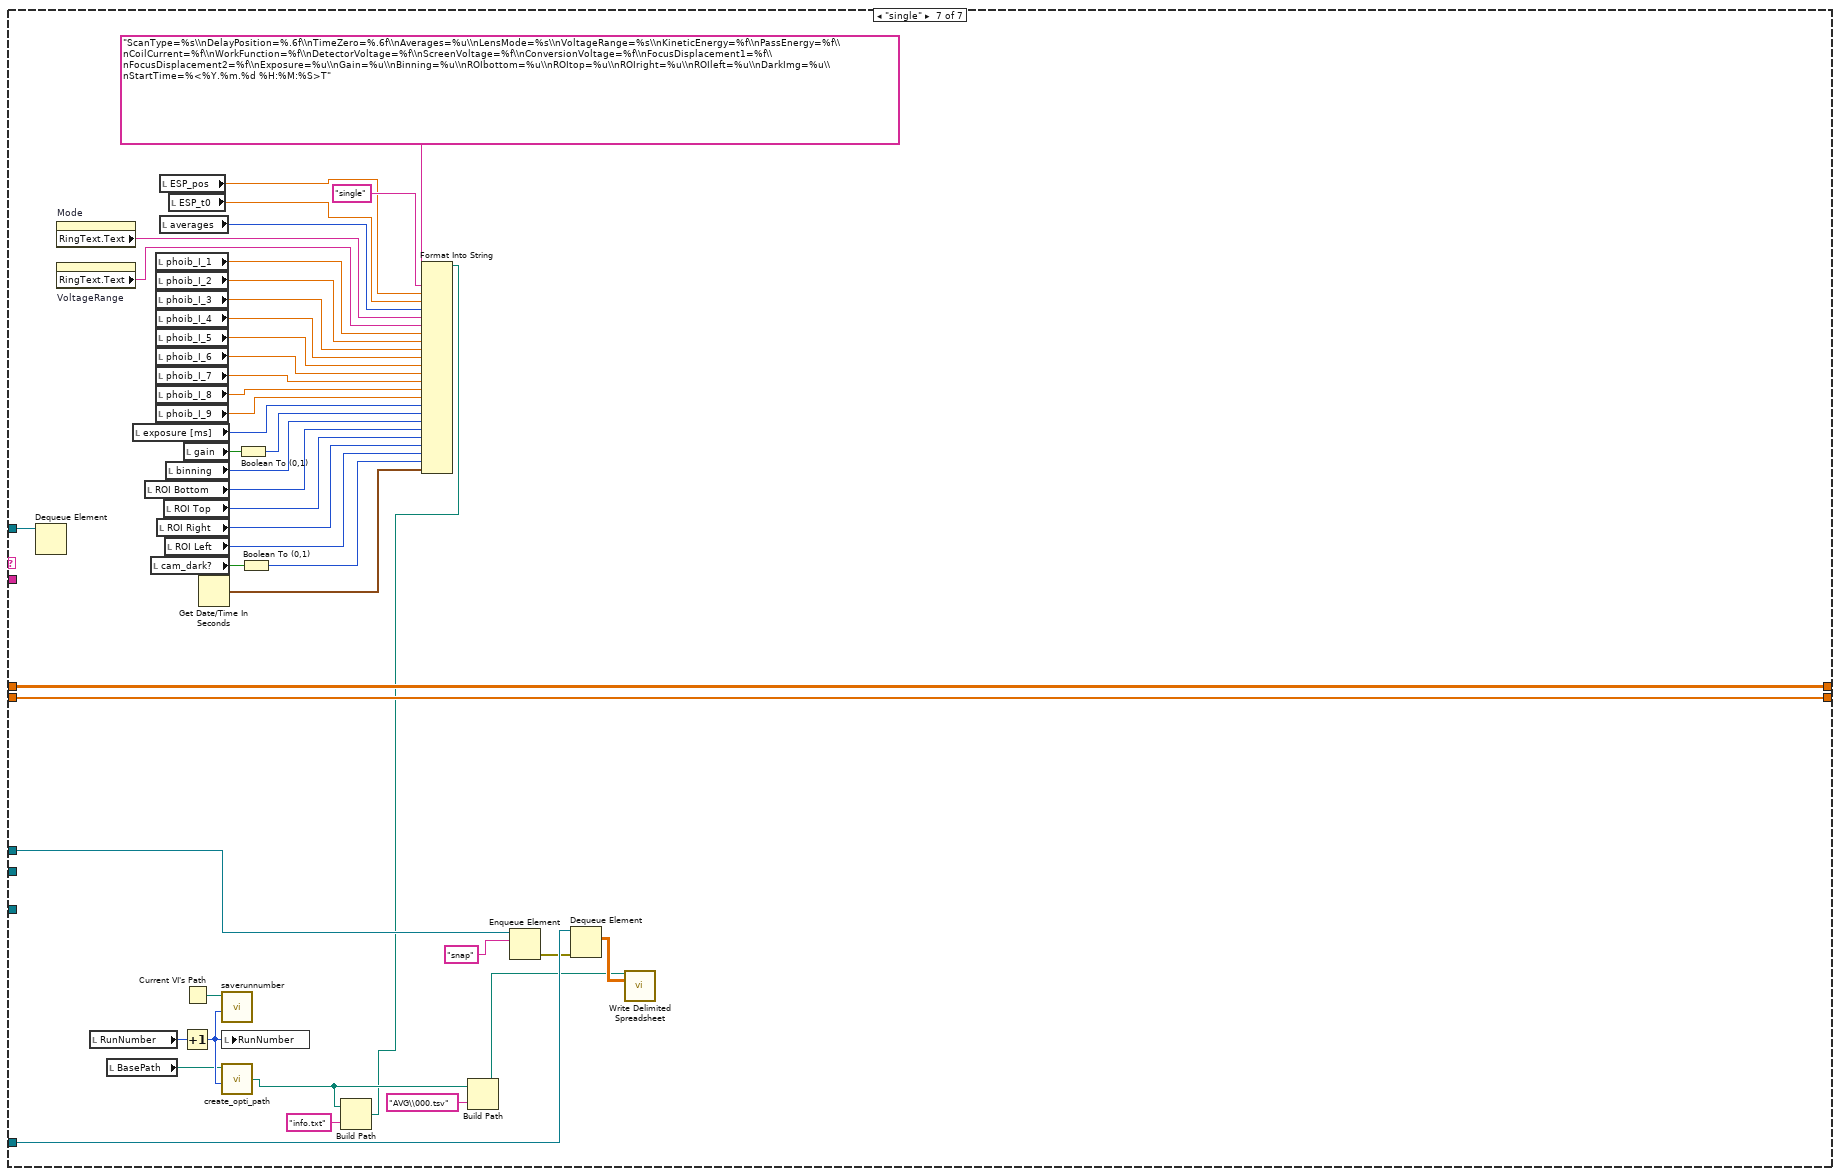
[diagram p9: hidden frame]
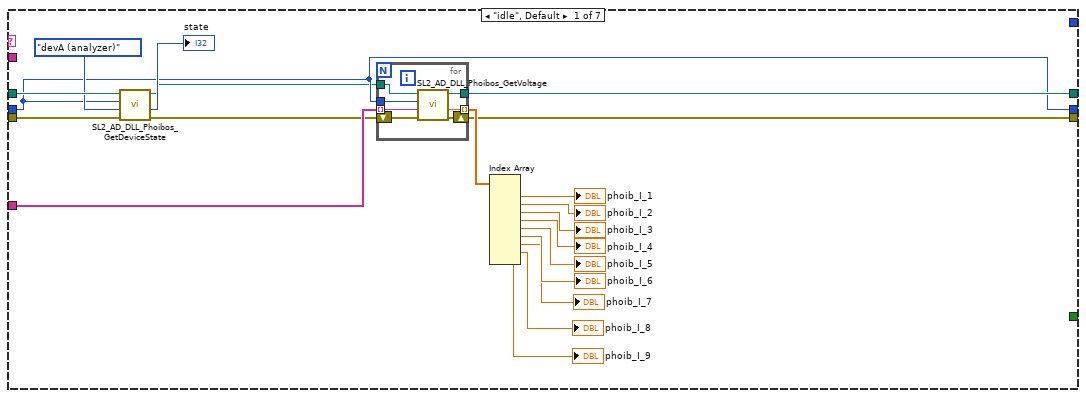
[diagram p10: hidden frame]
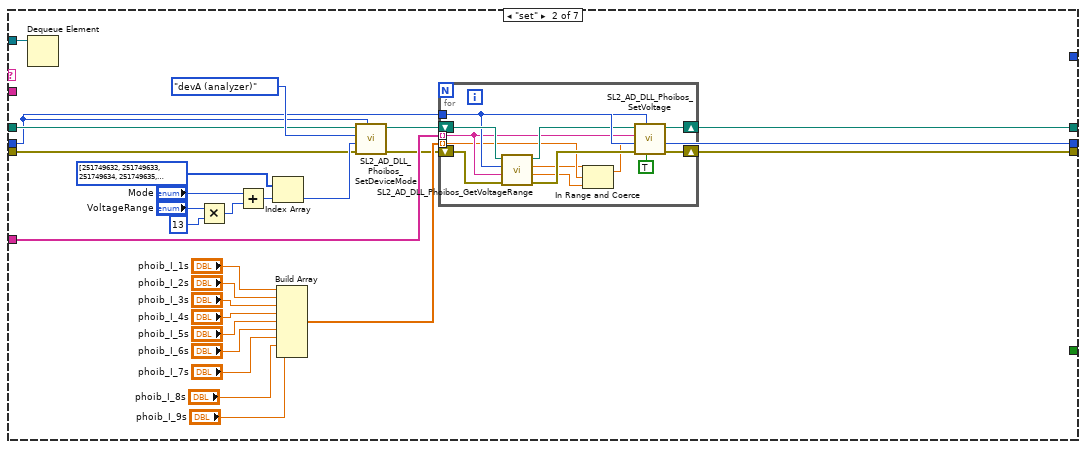
[diagram p11: hidden frame]
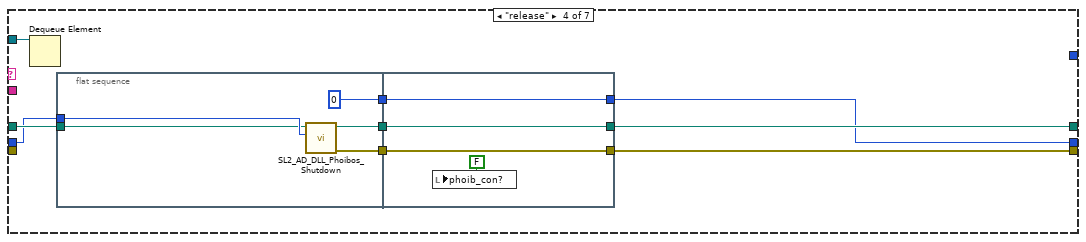
[diagram p12: hidden frame]
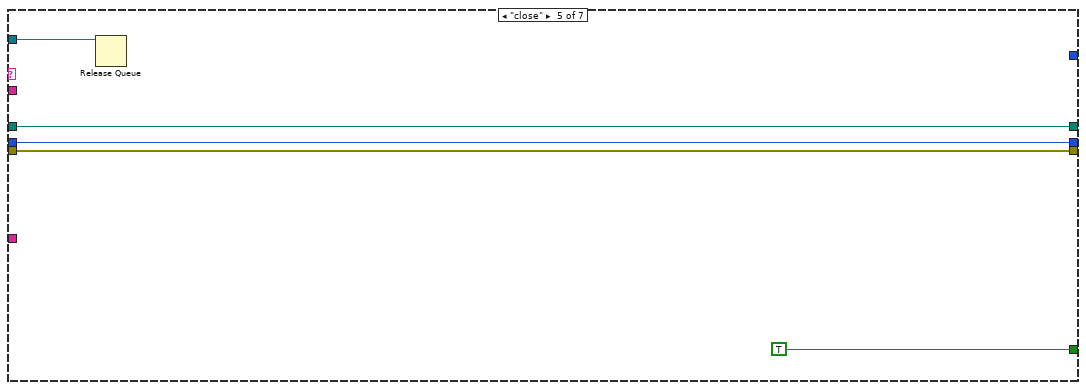
[diagram p13: hidden frame]
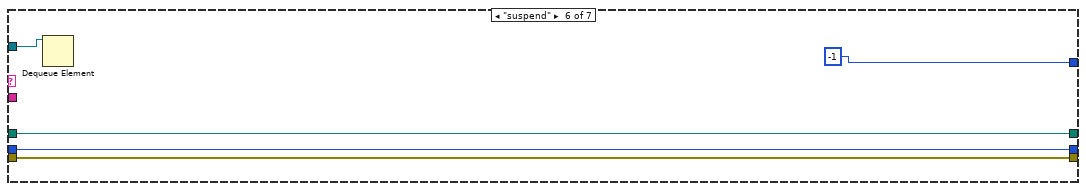
[diagram p14: hidden frame]
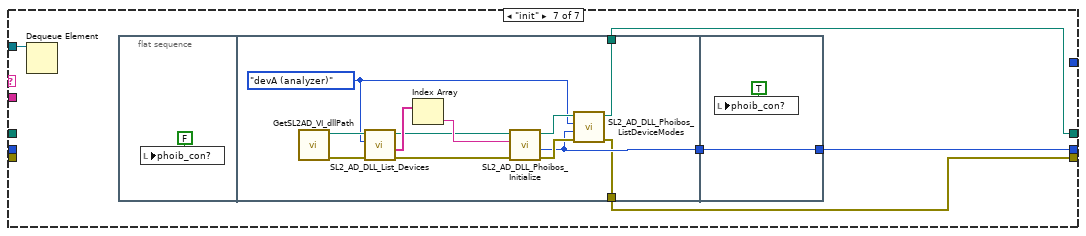
[diagram p15: hidden frame]
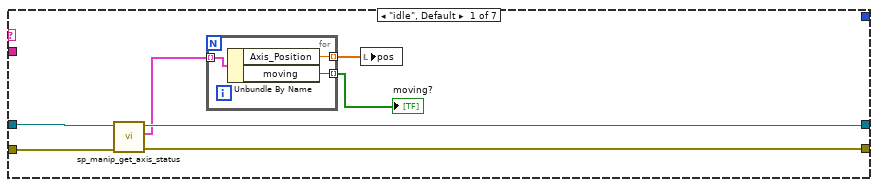
[diagram p16: hidden frame]
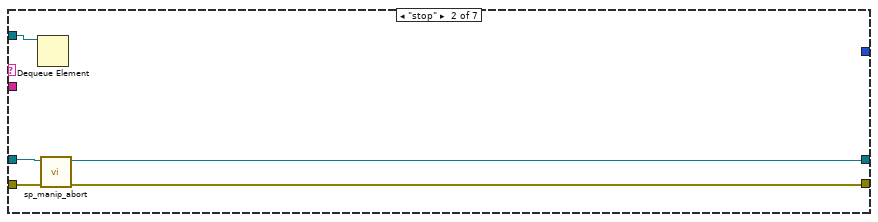
[diagram p17: hidden frame]
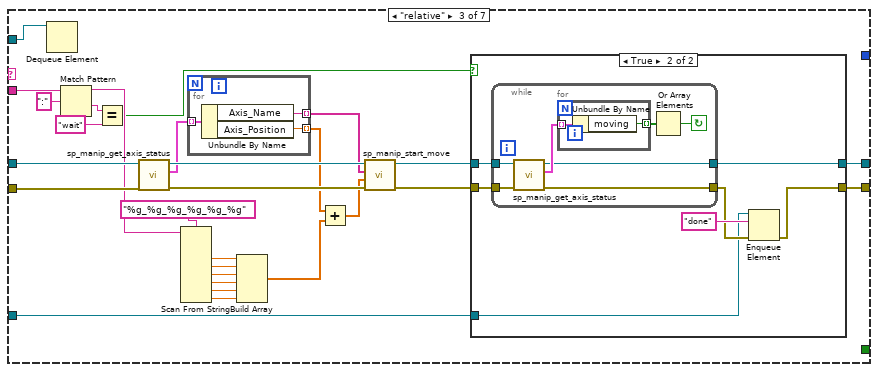
[diagram p18: hidden frame]
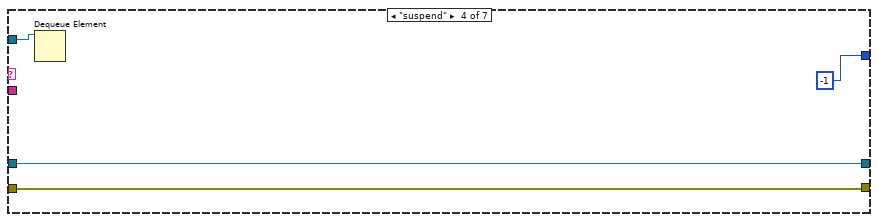
[diagram p20: hidden frame]
diagram:
  w14 = "init" ("name (unnamed)")
  w16 = "" ("name (unnamed)")
  # "scanvector"
  # "imgs"
  # "avg img"
  # "avg"
  # "time"
  # "dark"
  # "Error"
  # "Handle"
  # "memory pointer"
  n1 = Current VI's Path() -> (path=w4:path)
  n2 = Strip Path(path=w4) -> (stripped path=w8:path)  [unwired: 1 out]
  n3 = Strip Path(path=w8) -> (stripped path=w9:path)  [unwired: 1 out]
  n4 = Build Path(base path=w9, name or relative path="runnumber.txt") -> (appended path=w6:path)
  n5 = Obtain Queue(name (unnamed)="dataQ", element data type=dbl[][] []) -> (queue out=w11:refnum<queue>)  [unwired: 3 in, 2 out]
  n6 = Obtain Queue(name (unnamed)="cam", element data type=w16) -> (queue out=w36:refnum<queue>, error out=w35:errorcluster)  [unwired: 3 in, 1 out]
  n7 = Obtain Queue(name (unnamed)="ESP", element data type=w16) -> (queue out=w33:refnum<queue>, error out=w34:errorcluster)  [unwired: 3 in, 1 out]
  n8 = Obtain Queue(name (unnamed)="manip", element data type=w16) -> (queue out=w30:refnum<queue>, error out=w29:errorcluster)  [unwired: 3 in, 1 out]
  n9 = Obtain Queue(name (unnamed)="phoib", element data type=w16) -> (queue out=w27:refnum<queue>, error out=w28:errorcluster)  [unwired: 3 in, 1 out]
  n10 = Obtain Queue(name (unnamed)="meas", element data type=w16) -> (queue out=w2:refnum<queue>)  [unwired: 3 in, 2 out]
  n11 = Read from Text File(file (use dialog)=w6) -> (text=w7:string)  [unwired: 3 in, 3 out]
  n12 = Enqueue Element(queue=w36, element=w14, error in (no error)=w35) -> (queue out=w10:refnum<queue>)  [unwired: 1 in, 2 out]
  n13 = Enqueue Element(queue=w33, element=w14, error in (no error)=w34) -> (queue out=w13:refnum<queue>)  [unwired: 1 in, 2 out]
  n14 = Enqueue Element(queue=w30, element="suspend" ("name (unnamed)"), error in (no error)=w29) -> (queue out=w3:refnum<queue>)  [unwired: 1 in, 2 out]
  n15 = Enqueue Element(queue=w27, element=w14, error in (no error)=w28) -> (queue out=w24:refnum<queue>)  [unwired: 1 in, 2 out]
  n16 = Decimal String To Number(string=w7) -> (number=w1:i32)  [unwired: 2 in, 1 out]
  n17 = local write "RunNumber"(w1) -> ()
  n18 = while {
    tunnel: w11 -> [w52]
    tunnel: w13 -> [w51]
    tunnel: w10 -> [w50]
    shift-right: [w47] -> _
    shift-left: _ -> [w49]
    shift-right: [w46] -> _
    shift-left: _ -> [w48]
    tunnel: w2 -> [w43]
    tunnel: w3 -> [w38]
    stop <- w39 stop-if-true
    n19 = Preview Queue Element(queue=w43) -> (queue out=w40:refnum<queue>, element=w45:string)  [unwired: 2 in, 2 out]
    n20 = Match Pattern(string=w45, regular expression=":") -> (before substring=w42:string, after substring=w41:string)  [unwired: 1 in, 2 out]
    n21 = case shown="\"delay_chop\"" w42 {
      tunnel: w52 -> [_ _ w85 w242 _ w415 w520]
      tunnel: w51 -> [_ _ w84 w241 _ _ _]
      tunnel: w50 -> [_ _ w83 w240 _ w414 w522]
      tunnel: w49 -> [w54 w58 _ _ w376 w411 w519]
      tunnel: w48 -> [w53 w57 _ _ w374 w410 w518]
      tunnel: [w54 w58 w82 w239 w376 w411 w519] -> w47
      tunnel: [w53 w57 w65 w222 w374 w410 w518] -> w46
      tunnel: w41 -> [_ _ _ _ _ _ _]
      tunnel: w40 -> [w56 _ w74 w231 w378 w409 w521]
      tunnel: [TRUE _ _ _ _ _ _] -> w39
      tunnel: w38 -> [_ _ _ _ _ w413 _]
      frame "close" {
        n22 = Release Queue(queue=w56) -> ()  [unwired: 2 in, 3 out]
      }
      frame "idle", Default {
      }
      frame "GO" {
        n23 = Dequeue Element(queue=w74) -> (queue out=w73:refnum<queue>)  [unwired: 2 in, 3 out]
        n24 = local read "RunNumber"() -> (w80:u16)
        n25 = local read "BasePath"() -> (w79:path)
        n26 = local read "ESP Axis"() -> (w77:i32)
        n27 = local read "ESP_t0"() -> (w63:dbl)
        n28 = Increment(x=w80) -> (x+1=w78:u16)
        n29 = Current VI's Path() -> (path=w81:path)
        n30 = call "2delaypoints.vi"("Offset (mm)"=w63, "delay table [fs]"="delay table [fs]") -> ("delay points [mm]"=w62:dbl[], "delay pointss [fs]"=w60:dbl[])
        n31 = Number To Decimal String(number=w77) -> (decimal integer string=w76:string)  [unwired: 1 in]
        n32 = call "create_opti_path.vi"("RunNumber"=w78, "base path"=w79) -> ("Path"=w70:path)  [unwired: 2 in]
        n33 = call "saverunnumber.vi"("RunNumber"=w78, "VI path"=w81) -> ()  [unwired: 10 in]
        n34 = local write "RunNumber"(w78) -> ()
        n35 = Get Date/Time In Seconds() -> (seconds since 1Jan1904=w59:timestamp)
        n36 = Build Path(base path=w70, name or relative path="info.txt") -> (appended path=w61:path)
        n37 = while {
          tunnel: w62 -> [w122]
          tunnel: w76 -> [w130]
          tunnel: w84 -> [w129]
          tunnel: w85 -> [w128]
          tunnel: w73 -> [w127]
          tunnel: w83 -> [w126]
          tunnel: w70 -> [w125]
          shift-right: [w123] -> w82
          shift-left: dbl[][][] [] -> [w124]
          tunnel: [w121] -> w66
          tunnel: w61 -> [w88]
          tunnel: w60 -> [w87]
          tunnel: w59 -> [w86]
          i -> [w120]
          stop <- w116 stop-if-true
          n38 = for {
            N -> [w150]
            tunnel: w122 -> [w159] mode=indexing
            tunnel: w130 -> [w176]
            tunnel: w129 -> [w175]
            tunnel: w128 -> [w170]
            tunnel: w127 -> [w174]
            tunnel: w126 -> [w173]
            tunnel: w125 -> [w144]
            shift-right: [w134] -> w123
            shift-left: w124 -> [w166]
            tunnel: w120 -> [w143]
            tunnel: w87 -> [w132]
            tunnel: [w132] -> w121
            tunnel: [w156] -> w118
            tunnel: w86 -> [w146]
            tunnel: "delscan_iters" -> [w151]
            i -> [w136]
            stop <- "delscan_abort" stop-if-true
            w178 = ":" ("string")
            # "average data"
            # "init array?"
            n39 = Number To Fractional String(number=w159) -> (F-format string=w168:string)  [unwired: 3 in]
            n40 = property on="delscan_progress" class="Slide (strict)"("Scale.Maximum"=w150) -> ()  [unwired: 2 in, 2 out]
            n41 = Get Date/Time In Seconds() -> (seconds since 1Jan1904=w154:timestamp)
            n42 = call "createFileStruc.vi"("i_iter"=w143, "i_delay"=w136, "meas_path"=w144) -> ("AVG file"=w139:path, "RAW file"=w140:path)  [unwired: 7 in]
            n43 = Concatenate Strings("abs:" ("string"), w176, w178, w168, w178, "wait" ("string")) -> (w181:string)
            n44 = Enqueue Element(queue=w175, element=w181) -> (error out=w179:errorcluster)  [unwired: 2 in, 2 out]
            n45 = Subtract(x=w154, y=w146) -> (x-y=w152:dbl)
            n46 = Equal To 0?(x=w136) -> (x = 0?=w142:bool)
            n47 = Equal To 0?(x=w143) -> (x = 0?=w141:bool)
            n48 = Dequeue Element(queue=w174, error in (no error)=w179) -> (error out=w171:errorcluster)  [unwired: 1 in, 3 out]
            n49 = And(x=w142, y=w141) -> (x .and. y?=w167:bool)
            n50 = Enqueue Element(queue=w173, element="snap", error in (no error)=w171) -> (error out=w169:errorcluster)  [unwired: 1 in, 2 out]
            n51 = Dequeue Element(queue=w170, error in (no error)=w169) -> (element=w162:dbl[][])  [unwired: 1 in, 3 out]
            n52 = Multiply(x=w150, y=w143) -> (x*y=w155:i32)
            n53 = Multiply(x=w150, y=w151) -> (x*y=w149:u32)
            n54 = Array Size(array=w162) -> (size(s)=w163:i32[])
            n55 = Add(x=w155, y=w136) -> (x+y=w153:i32)
            n56 = call-poly <vilib>:"Write Delimited Spreadsheet.vi"("file path (dialog if empty)"=w140, "2D data"=w162) -> ()  [unwired: 12 in, 2 out]
            n57 = Index Array(array=w163) -> (element #1=w161:i32, element #2=w160:i32)  [unwired: 2 in]
            n58 = Divide(x=w152, y=w153) -> (x/y=w148:dbl)
            "time / step" <- w148
            n59 = Multiply(x=w149, y=w148) -> (x*y=w147:dbl)
            n60 = case shown="True" w167 {
              tunnel: w150 -> [_ w189]
              tunnel: [w184 w187] -> w165
              tunnel: w166 -> [w184 _]
              tunnel: w161 -> [_ w186]
              tunnel: w160 -> [_ w185]
              frame False {
              }
              frame True {
                n61 = Initialize Array(0.0 ("element"), w189, w186, w185) -> (w187:dbl[][][])
              }
            }
            n62 = Add(x=w146, y=w147) -> (x+y=→"del_ETA":timestamp)
            n63 = for {
              N: w161 -> [_]
              tunnel: w136 -> [w196]
              shift-right: [w194] -> w134
              shift-left: w165 -> [w197]
              tunnel: w143 -> [w192]
              shift-right: [w191] -> w164
              shift-left: w162 -> [w193]
              tunnel: w160 -> [w190]
              i -> [w195]
              n64 = for {
                N: w190 -> [_]
                tunnel: w196 -> [w204]
                tunnel: w195 -> [w201]
                shift-right: [w203] -> w194
                shift-left: w197 -> [w205]
                tunnel: w192 -> [w199]
                shift-right: [w198] -> w191
                shift-left: w193 -> [w202]
                i -> [w200]
                n65 = in-place {
                  in-place-border: w199 -> [w211]
                  n66 = in-place-array #1(w205, w204, w201, w200) -> (w212:dbl)
                  n67 = in-place-array #2(w202, w201, w200) -> (w209:dbl)
                  n68 = Multiply(x=w212, y=w211) -> (x*y=w210:dbl)
                  n69 = Increment(x=w211) -> (x+1=w207:i32)
                  n70 = Add(x=w210, y=w209) -> (x+y=w208:dbl)
                  n71 = Divide(x=w208, y=w207) -> (x/y=w206:dbl)
                  n72 = in-place-array #1(w206) -> (w203:dbl[][][])  [unwired: 3 out]
                  n73 = in-place-array #2(w206) -> (w198:dbl[][])  [unwired: 2 out]
                }
              }
            }
            n74 = call-poly <vilib>:"Write Delimited Spreadsheet.vi"("file path (dialog if empty)"=w139, "2D data"=w164) -> ()  [unwired: 12 in, 2 out]
            n75 = property on="mainimg" class="IntGraph (strict)"() -> ("CrsrLis"=w135:T4)  [unwired: 2 in, 2 out]
            n76 = call "processData.vi"("Cursor List"=w135, "data in"=w134) -> ("Intensity Chart"=w133:dbl[])  [unwired: 1 in, 2 out]
            n77 = Increment(x=w136) -> (x+1=w137:i32)
            n78 = Bundle("delay pointss [fs]"=w132, "Intensity Chart"=w133) -> (w131:T5)  [unwired: 1 in]
            n79 = flat-sequence {
              tunnel: w131 -> [w183]
              tunnel: [w183] -> w138
              tunnel: w137 -> [w182]
              frame #0 {
                "delscan_progress" <- w182
              }
            }
            n80 = Or(x="delscan_finishIteration", y="delscan_abort") -> (x .or. y?=w156:bool)
            "delscan_pos" <- w159
            "scangraph" <- w138
          }
          n81 = Increment(x=w120) -> (x+1=w119:i32)
          "iteration" <- w119
          n82 = local read "exposure [ms]"() -> (w103:u32)
          n83 = local read "delscan_iters"() -> (w113:u32)
          n84 = local read "ROI Bottom"() -> (w106:i32)
          n85 = property on="Mode" class="Enum (strict)"() -> ("RingText.Text"=w92:string)  [unwired: 2 in, 2 out]
          n86 = property on="VoltageRange" class="Enum (strict)"() -> ("RingText.Text"=w93:string)  [unwired: 2 in, 2 out]
          n87 = local read "cam_dark?"() -> (w90:bool)
          n88 = local read "phoib_I_1"() -> (w94:dbl)
          n89 = local read "phoib_I_2"() -> (w95:dbl)
          n90 = local read "phoib_I_3"() -> (w96:dbl)
          n91 = local read "phoib_I_4"() -> (w97:dbl)
          n92 = local read "phoib_I_5"() -> (w98:dbl)
          n93 = local read "phoib_I_6"() -> (w99:dbl)
          n94 = local read "phoib_I_7"() -> (w100:dbl)
          n95 = local read "phoib_I_8"() -> (w101:dbl)
          n96 = local read "phoib_I_9"() -> (w102:dbl)
          n97 = local read "ROI Right"() -> (w108:i32)
          n98 = local read "averages"() -> (w112:i32)
          n99 = local read "ROI Top"() -> (w107:i32)
          n100 = local read "ROI Left"() -> (w109:i32)
          n101 = local read "binning"() -> (w105:u16)
          n102 = local read "ESP_t0"() -> (w114:dbl)
          n103 = local read "gain"() -> (w89:bool)
          n104 = Boolean To (0,1)(Boolean=w89) -> (0, 1=w104:i16)
          n105 = Boolean To (0,1)(Boolean=w90) -> (0, 1=w110:i16)
          n106 = Format Into String(format string="ScanType:%s\\nAverages:%u\\nRepetitions:%u\\nTimeZero:%f\\nLensMode:%s\\nVoltageRange:%s\\nKineticEnergy:%f\\nPassEnergy:%f\\nCoilCurrent:%f\\nWorkFunction:%f\\nDetectorVoltage:%f\\nScreenVoltage:%f\\nConversionVoltage:%f\\nFocusDisplacement1:%f\\nFocusDisplacement2:%f\\nExposure:%u\\nGain:%u\\nBinning:%u\\nROIbottom:%u\\nROItop:%u\\nROIright:%u\\nROIleft:%u\\nDarkImg:%u\\nStartTime:%<%Y.%m.%d %H:%M:%S>T", initial string=w88, "delay" ("input 1"), w112, w113, w114, w92, w93, w94, w95, w96, w97, w98, w99, w100, w101, w102, w103, w104, w105, w106, w107, w108, w109, w110, w86) -> ()  [unwired: 1 in, 2 out]
          n107 = Less Or Equal?(x="delscan_iters", y=w119) -> (x <= y?=w117:bool)
          n108 = Or(x=w118, y=w117) -> (x .or. y?=w116:bool)
        }
        n109 = Build Path(base path=w70, name or relative path="scanvector.txt") -> (appended path=w67:path)
        n110 = call-poly <vilib>:"Write Delimited Spreadsheet.vi"("file path (dialog if empty)"=w67, "format (%.3f)"="%.6f", "1D data"=w62, "transpose? (F)"=TRUE) -> ()  [unwired: 10 in, 2 out]
        n111 = flat-sequence {
          tunnel: w66 -> [w215]
          tunnel: [w215] -> w65
          frame #0 {
            w214 = u32 1000 ("frequency (Hz)")
            n112 = call <vilib>:"Beep.vi"("use system alert? (T)"=FALSE, "duration (msec)"=w214, "frequency (Hz)"=w214) -> ()  [unwired: 9 in]
          }
        }
      }
      frame "delay_chop" {
        n113 = local read "delay table [fs]"() -> (w216:string[][])
        n114 = Dequeue Element(queue=w231) -> (queue out=w230:refnum<queue>)  [unwired: 2 in, 3 out]
        n115 = local read "RunNumber"() -> (w237:u16)
        n116 = local read "BasePath"() -> (w236:path)
        n117 = local read "ESP Axis"() -> (w234:i32)
        n118 = local read "ESP_t0"() -> (w221:dbl)
        n119 = Increment(x=w237) -> (x+1=w235:u16)
        n120 = Current VI's Path() -> (path=w238:path)
        n121 = call "2delaypoints.vi"("Offset (mm)"=w221, "delay table [fs]"=w216) -> ("delay points [mm]"=w220:dbl[], "delay pointss [fs]"=w218:dbl[])
        n122 = Number To Decimal String(number=w234) -> (decimal integer string=w233:string)  [unwired: 1 in]
        n123 = call "create_opti_path.vi"("RunNumber"=w235, "base path"=w236) -> ("Path"=w227:path)  [unwired: 2 in]
        n124 = call "saverunnumber.vi"("RunNumber"=w235, "VI path"=w238) -> ()  [unwired: 10 in]
        n125 = local write "RunNumber"(w235) -> ()
        n126 = Get Date/Time In Seconds() -> (seconds since 1Jan1904=w217:timestamp)
        n127 = Build Path(base path=w227, name or relative path="info.txt") -> (appended path=w219:path)
        n128 = while {
          tunnel: w220 -> [w279]
          tunnel: w233 -> [w287]
          tunnel: w241 -> [w286]
          tunnel: w242 -> [w285]
          tunnel: w230 -> [w284]
          tunnel: w240 -> [w283]
          tunnel: w227 -> [w282]
          shift-right: [w280] -> w239
          shift-left: dbl[][][] [] -> [w281]
          tunnel: [w278] -> w223
          tunnel: w219 -> [w247]
          tunnel: w218 -> [w246]
          tunnel: w217 -> [w245]
          i -> [w277]
          stop <- w274 stop-if-true
          n129 = Increment(x=w277) -> (x+1=w244:i32)
          n130 = local read "exposure [ms]"() -> (w262:u32)
          n131 = local read "delscan_iters"() -> (w272:u32)
          n132 = local read "ROI Bottom"() -> (w265:i32)
          n133 = property on="Mode" class="Enum (strict)"() -> ("RingText.Text"=w251:string)  [unwired: 2 in, 2 out]
          n134 = property on="VoltageRange" class="Enum (strict)"() -> ("RingText.Text"=w252:string)  [unwired: 2 in, 2 out]
          n135 = local read "cam_dark?"() -> (w249:bool)
          n136 = local write "iteration"(w244) -> ()
          n137 = local read "phoib_I_1"() -> (w253:dbl)
          n138 = local read "phoib_I_2"() -> (w254:dbl)
          n139 = local read "phoib_I_3"() -> (w255:dbl)
          n140 = local read "phoib_I_4"() -> (w256:dbl)
          n141 = local read "phoib_I_5"() -> (w257:dbl)
          n142 = local read "phoib_I_6"() -> (w258:dbl)
          n143 = local read "phoib_I_7"() -> (w259:dbl)
          n144 = local read "phoib_I_8"() -> (w260:dbl)
          n145 = local read "phoib_I_9"() -> (w261:dbl)
          n146 = local read "ROI Right"() -> (w267:i32)
          n147 = local read "averages"() -> (w271:i32)
          n148 = local read "ROI Top"() -> (w266:i32)
          n149 = local read "ROI Left"() -> (w268:i32)
          n150 = local read "binning"() -> (w264:u16)
          n151 = local read "ESP_t0"() -> (w273:dbl)
          n152 = local read "gain"() -> (w248:bool)
          n153 = Boolean To (0,1)(Boolean=w248) -> (0, 1=w263:i16)
          n154 = Boolean To (0,1)(Boolean=w249) -> (0, 1=w269:i16)
          n155 = local read "delscan_iters"() -> (w243:u32)
          n156 = for {
            N -> [w294]
            tunnel: w279 -> [w291] mode=indexing
            tunnel: w287 -> [w333]
            tunnel: w286 -> [w332]
            tunnel: w285 -> [w327]
            tunnel: w284 -> [w331]
            tunnel: w283 -> [w330]
            tunnel: w282 -> [w307]
            shift-right: [w298] -> w280
            shift-left: w281 -> [w323]
            tunnel: w277 -> [w306]
            tunnel: w246 -> [w296]
            tunnel: [w296] -> w278
            tunnel: [w316] -> w276
            tunnel: w245 -> [w308]
            tunnel: w243 -> [w311]
            i -> [w300]
            stop <- "delscan_abort 2" stop-if-true
            w335 = ":" ("string")
            # "average data"
            # "init array?"
            n157 = local write "delscan_pos"(w291) -> ()
            n158 = Number To Fractional String(number=w291) -> (F-format string=w325:string)  [unwired: 3 in]
            n159 = Get Date/Time In Seconds() -> (seconds since 1Jan1904=w314:timestamp)
            n160 = call "createFileStruc.vi"("i_iter"=w306, "i_delay"=w300, "meas_path"=w307) -> ("AVG file"=w302:path, "RAW file"=w303:path)  [unwired: 7 in]
            n161 = property on="delscan_progress" class="Slide (strict)"("Scale.Maximum"=w294) -> ()  [unwired: 2 in, 2 out]
            n162 = Concatenate Strings("abs:" ("string"), w333, w335, w325, w335, "wait" ("string")) -> (w338:string)
            n163 = Enqueue Element(queue=w332, element=w338) -> (error out=w336:errorcluster)  [unwired: 2 in, 2 out]
            n164 = Subtract(x=w314, y=w308) -> (x-y=w312:dbl)
            n165 = Equal To 0?(x=w300) -> (x = 0?=w305:bool)
            n166 = Equal To 0?(x=w306) -> (x = 0?=w304:bool)
            n167 = Dequeue Element(queue=w331, error in (no error)=w336) -> (error out=w328:errorcluster)  [unwired: 1 in, 3 out]
            n168 = And(x=w305, y=w304) -> (x .and. y?=w324:bool)
            n169 = Enqueue Element(queue=w330, element="snap", error in (no error)=w328) -> (error out=w326:errorcluster)  [unwired: 1 in, 2 out]
            n170 = Dequeue Element(queue=w327, error in (no error)=w326) -> (element=w319:dbl[][])  [unwired: 1 in, 3 out]
            n171 = Multiply(x=w294, y=w306) -> (x*y=w315:i32)
            n172 = Multiply(x=w294, y=w311) -> (x*y=w310:u32)
            n173 = Array Size(array=w319) -> (size(s)=w320:i32[])
            n174 = Add(x=w315, y=w300) -> (x+y=w313:i32)
            n175 = call-poly <vilib>:"Write Delimited Spreadsheet.vi"("file path (dialog if empty)"=w303, "2D data"=w319) -> ()  [unwired: 12 in, 2 out]
            n176 = Index Array(array=w320) -> (element #1=w318:i32, element #2=w317:i32)  [unwired: 2 in]
            n177 = Divide(x=w312, y=w313) -> (x/y=w292:dbl)
            n178 = Multiply(x=w310, y=w292) -> (x*y=w309:dbl)
            n179 = case shown="True" w324 {
              tunnel: w294 -> [_ w346]
              tunnel: [w341 w344] -> w322
              tunnel: w323 -> [w341 _]
              tunnel: w318 -> [_ w343]
              tunnel: w317 -> [_ w342]
              frame False {
              }
              frame True {
                n180 = Initialize Array(0.0 ("element"), w346, w343, w342) -> (w344:dbl[][][])
              }
            }
            n181 = Add(x=w308, y=w309) -> (x+y=w293:timestamp)
            n182 = local write "del_ETA"(w293) -> ()
            n183 = local write "time / step"(w292) -> ()
            n184 = for {
              N: w318 -> [_]
              tunnel: w300 -> [w353]
              shift-right: [w351] -> w298
              shift-left: w322 -> [w354]
              tunnel: w306 -> [w349]
              shift-right: [w348] -> w321
              shift-left: w319 -> [w350]
              tunnel: w317 -> [w347]
              i -> [w352]
              n185 = for {
                N: w347 -> [_]
                tunnel: w353 -> [w361]
                tunnel: w352 -> [w358]
                shift-right: [w360] -> w351
                shift-left: w354 -> [w362]
                tunnel: w349 -> [w356]
                shift-right: [w355] -> w348
                shift-left: w350 -> [w359]
                i -> [w357]
                n186 = in-place {
                  in-place-border: w356 -> [w368]
                  n187 = in-place-array #3(w362, w361, w358, w357) -> (w369:dbl)
                  n188 = in-place-array #4(w359, w358, w357) -> (w366:dbl)
                  n189 = Multiply(x=w369, y=w368) -> (x*y=w367:dbl)
                  n190 = Increment(x=w368) -> (x+1=w364:i32)
                  n191 = Add(x=w367, y=w366) -> (x+y=w365:dbl)
                  n192 = Divide(x=w365, y=w364) -> (x/y=w363:dbl)
                  n193 = in-place-array #3(w363) -> (w360:dbl[][][])  [unwired: 3 out]
                  n194 = in-place-array #4(w363) -> (w355:dbl[][])  [unwired: 2 out]
                }
              }
            }
            n195 = call-poly <vilib>:"Write Delimited Spreadsheet.vi"("file path (dialog if empty)"=w302, "2D data"=w321) -> ()  [unwired: 12 in, 2 out]
            n196 = property on="mainimg" class="IntGraph (strict)"() -> ("CrsrLis"=w299:T4)  [unwired: 2 in, 2 out]
            n197 = call "processData.vi"("Cursor List"=w299, "data in"=w298) -> ("Intensity Chart"=w297:dbl[])  [unwired: 1 in, 2 out]
            n198 = Increment(x=w300) -> (x+1=w301:i32)
            n199 = Bundle("delay pointss [fs]"=w296, "Intensity Chart"=w297) -> (w295:T5)  [unwired: 1 in]
            n200 = flat-sequence {
              tunnel: w295 -> [w340]
              tunnel: [w340] -> w290
              tunnel: w301 -> [w339]
              frame #0 {
                n201 = local write "delscan_progress"(w339) -> ()
              }
            }
            n202 = Or(x="delscan_finishIteration 2", y="delscan_abort 2") -> (x .or. y?=w316:bool)
            n203 = local write "scangraph"(w290) -> ()
          }
          n204 = Format Into String(format string="ScanType:%s\\nAverages:%u\\nRepetitions:%u\\nTimeZero:%f\\nLensMode:%s\\nVoltageRange:%s\\nKineticEnergy:%f\\nPassEnergy:%f\\nCoilCurrent:%f\\nWorkFunction:%f\\nDetectorVoltage:%f\\nScreenVoltage:%f\\nConversionVoltage:%f\\nFocusDisplacement1:%f\\nFocusDisplacement2:%f\\nExposure:%u\\nGain:%u\\nBinning:%u\\nROIbottom:%u\\nROItop:%u\\nROIright:%u\\nROIleft:%u\\nDarkImg:%u\\nStartTime:%<%Y.%m.%d %H:%M:%S>T", initial string=w247, "delay" ("input 1"), w271, w272, w273, w251, w252, w253, w254, w255, w256, w257, w258, w259, w260, w261, w262, w263, w264, w265, w266, w267, w268, w269, w245) -> ()  [unwired: 1 in, 2 out]
          n205 = Less Or Equal?(x=w243, y=w244) -> (x <= y?=w275:bool)
          n206 = Or(x=w276, y=w275) -> (x .or. y?=w274:bool)
        }
        n207 = Build Path(base path=w227, name or relative path="scanvector.txt") -> (appended path=w224:path)
        n208 = call-poly <vilib>:"Write Delimited Spreadsheet.vi"("file path (dialog if empty)"=w224, "format (%.3f)"="%.6f", "1D data"=w220, "transpose? (F)"=TRUE) -> ()  [unwired: 10 in, 2 out]
        n209 = flat-sequence {
          tunnel: w223 -> [w372]
          tunnel: [w372] -> w222
          frame #0 {
            w371 = u32 1000 ("frequency (Hz)")
            n210 = call <vilib>:"Beep.vi"("use system alert? (T)"=FALSE, "duration (msec)"=w371, "frequency (Hz)"=w371) -> ()  [unwired: 9 in]
          }
        }
      }
      frame "refresh" {
        n211 = Dequeue Element(queue=w378) -> ()  [unwired: 2 in, 4 out]
        n212 = property on="mainimg" class="IntGraph (strict)"() -> ("CrsrLis"=w377:T4)  [unwired: 2 in, 2 out]
        n213 = call "processData.vi"("Cursor List"=w377, "data in"=w376) -> ("Intensity Chart"=w375:dbl[])  [unwired: 1 in, 2 out]
        n214 = Bundle("delay pointss [fs]"=w374, "Intensity Chart"=w375) -> (w373:T5)  [unwired: 1 in]
        n215 = local write "scangraph"(w373) -> ()
      }
      frame "manip" {
        n216 = Dequeue Element(queue=w409) -> (queue out=w408:refnum<queue>)  [unwired: 2 in, 3 out]
        n217 = local read "RunNumber"() -> (w417:u16)
        n218 = local read "BasePath"() -> (w418:path)
        n219 = property on="delscan_progress 2" class="Slide (strict)"("Scale.Maximum"="manip_scan_steps") -> ()  [unwired: 2 in, 2 out]
        n220 = Index Array(array="manip_scan_delta") -> (element #1=w430:dbl, element #2=w429:dbl, element #3=w428:dbl, element #4=w427:dbl, element #5=w426:dbl, element #6=w425:dbl)  [unwired: 6 in]
        n221 = Increment(x=w417) -> (x+1=w419:u16)
        n222 = Current VI's Path() -> (path=w416:path)
        n223 = Format Into String(format string="%g_%g_%g_%g_%g_%g", w430, w429, w428, w427, w426, w425) -> (resulting string=w423:string)  [unwired: 2 in, 1 out]
        n224 = property on="Mode" class="Enum (strict)"() -> ("RingText.Text"=w403:string)  [unwired: 2 in, 2 out]
        n225 = property on="VoltageRange" class="Enum (strict)"() -> ("RingText.Text"=w402:string)  [unwired: 2 in, 2 out]
        n226 = call "saverunnumber.vi"("RunNumber"=w419, "VI path"=w416) -> ()  [unwired: 10 in]
        n227 = local write "RunNumber"(w419) -> ()
        n228 = call "create_opti_path.vi"("RunNumber"=w419, "base path"=w418) -> ("Path"=w382:path)  [unwired: 2 in]
        n229 = local read "exposure [ms]"() -> (w392:u32)
        n230 = Build Path(base path=w382, name or relative path="info.txt") -> (appended path=w381:path)
        n231 = Concatenate Strings("relative:" ("string"), w423, ":wait" ("string")) -> (w432:string)
        n232 = local read "ROI Bottom"() -> (w389:i32)
        n233 = local read "cam_dark?"() -> (w406:bool)
        n234 = local read "phoib_I_1"() -> (w401:dbl)
        n235 = local read "phoib_I_2"() -> (w400:dbl)
        n236 = local read "phoib_I_3"() -> (w399:dbl)
        n237 = local read "phoib_I_4"() -> (w398:dbl)
        n238 = local read "phoib_I_5"() -> (w397:dbl)
        n239 = local read "phoib_I_6"() -> (w396:dbl)
        n240 = local read "phoib_I_7"() -> (w395:dbl)
        n241 = local read "phoib_I_8"() -> (w394:dbl)
        n242 = local read "phoib_I_9"() -> (w393:dbl)
        n243 = local read "ROI Right"() -> (w387:i32)
        n244 = local read "averages"() -> (w404:i32)
        n245 = local read "ROI Top"() -> (w388:i32)
        n246 = local read "ROI Left"() -> (w386:i32)
        n247 = local read "binning"() -> (w390:u16)
        n248 = local read "gain"() -> (w407:bool)
        n249 = Get Date/Time In Seconds() -> (seconds since 1Jan1904=w384:timestamp)
        n250 = Build Path(base path=w382, name or relative path="scanvector.txt") -> (appended path=w433:path)
        n251 = for {
          N: 1 -> [_]
          tunnel: w415 -> [w448]
          tunnel: w382 -> [w447]
          tunnel: w433 -> [w440]
          tunnel: "manip_scan_steps" -> [w439]
          tunnel: w432 -> [w438]
          tunnel: w413 -> [w437]
          tunnel: w408 -> [w436]
          tunnel: w414 -> [w435]
          tunnel: "manip_scan_delta" -> [w434]
          i -> [w442]
          n252 = Add(x=w442, y=1000) -> (x+y=w445:i32)
          n253 = Number To Decimal String(number=w445) -> (decimal integer string=w444:string)  [unwired: 1 in]
          n254 = String Subset(string=w444, offset (0)=1) -> (substring=w441:string)  [unwired: 1 in]
          n255 = for {
            N: w439 -> [_]
            tunnel: w448 -> [w471]
            tunnel: w447 -> [w468]
            tunnel: w441 -> [w462]
            tunnel: w440 -> [w464]
            tunnel: w438 -> [w459]
            tunnel: w437 -> [w458]
            tunnel: w436 -> [w457]
            tunnel: w435 -> [w456]
            tunnel: w434 -> [w454]
            i -> [w449]
            stop <- "abort" stop-if-true
            n256 = Increment(x=w449) -> (x+1=→"delscan_progress 2":i32)
            n257 = Multiply(x=w454, y=w449) -> (x*y=w453:dbl[])
            n258 = Enqueue Element(queue=w458, element=w459) -> (error out=w460:errorcluster)  [unwired: 2 in, 2 out]
            n259 = Add(x=w449, y=10000) -> (x+y=w477:i32)
            n260 = Dequeue Element(queue=w457, error in (no error)=w460) -> (error out=w455:errorcluster)  [unwired: 1 in, 3 out]
            n261 = Number To Decimal String(number=w477) -> (decimal integer string=w476:string)  [unwired: 1 in]
            n262 = String Subset(string=w476, offset (0)=1) -> (substring=w461:string)  [unwired: 1 in]
            n263 = Enqueue Element(queue=w456, element="snap", error in (no error)=w455) -> (error out=w470:errorcluster)  [unwired: 1 in, 2 out]
            n264 = Concatenate Strings("RAW\\" ("string"), w462, "_" ("string"), w461, ".tsv" ("string")) -> (w467:string)
            n265 = Dequeue Element(queue=w471, error in (no error)=w470) -> (element=w466:dbl[][])  [unwired: 1 in, 3 out]
            n266 = Build Path(base path=w468, name or relative path=w467) -> (appended path=w469:path)
            n267 = call-poly <vilib>:"Write Delimited Spreadsheet.vi"("file path (dialog if empty)"=w469, "2D data"=w466) -> ()  [unwired: 12 in, 2 out]
            n268 = call-poly <vilib>:"Write Delimited Spreadsheet.vi"("file path (dialog if empty)"=w464, "1D data"=w453, "append to file? (F)"=TRUE, "transpose? (F)"=FALSE) -> ()  [unwired: 10 in, 2 out]
          }
        }
        n269 = Boolean To (0,1)(Boolean=w407) -> (0, 1=w391:i16)
        n270 = Boolean To (0,1)(Boolean=w406) -> (0, 1=w385:i16)
        n271 = Format Into String(format string="ScanType:%s\\nAverages:%u\\nMode:%s\\nVoltageRange:%s\\nKineticEnergy:%f\\nPassEnergy:%f\\nCoilCurrent:%f\\nWorkFunction:%f\\nDetectorVoltage:%f\\nScreenVoltage:%f\\nConversionVoltage:%f\\nFocusDisplacement1:%f\\nFocusDisplacement2:%f\\nExposure:%u\\nGain:%u\\nBinning:%u\\nROIbottom:%u\\nROItop:%u\\nROIright:%u\\nROIleft:%u\\nDarkImg:%u\\nStartTime:%<%Y.%m.%d %H:%M:%S>T", initial string=w381, "manipulator" ("input 1"), w404, w403, w402, w401, w400, w399, w398, w397, w396, w395, w394, w393, w392, w391, w390, w389, w388, w387, w386, w385, w384) -> ()  [unwired: 1 in, 2 out]
      }
      frame "single" {
        n272 = Dequeue Element(queue=w521) -> ()  [unwired: 2 in, 4 out]
        n273 = property on="Mode" class="Enum (strict)"() -> ("RingText.Text"=w506:string)  [unwired: 2 in, 2 out]
        n274 = property on="VoltageRange" class="Enum (strict)"() -> ("RingText.Text"=w505:string)  [unwired: 2 in, 2 out]
        n275 = local read "RunNumber"() -> (w512:u16)
        n276 = local read "BasePath"() -> (w513:path)
        n277 = local read "exposure [ms]"() -> (w495:u32)
        n278 = local read "ROI Bottom"() -> (w492:i32)
        n279 = local read "cam_dark?"() -> (w509:bool)
        n280 = local read "phoib_I_1"() -> (w504:dbl)
        n281 = local read "phoib_I_2"() -> (w503:dbl)
        n282 = local read "phoib_I_3"() -> (w502:dbl)
        n283 = local read "phoib_I_4"() -> (w501:dbl)
        n284 = local read "phoib_I_5"() -> (w500:dbl)
        n285 = local read "phoib_I_6"() -> (w499:dbl)
        n286 = local read "phoib_I_7"() -> (w498:dbl)
        n287 = local read "phoib_I_8"() -> (w497:dbl)
        n288 = local read "phoib_I_9"() -> (w496:dbl)
        n289 = local read "ROI Right"() -> (w490:i32)
        n290 = local read "ESP_pos"() -> (w479:dbl)
        n291 = local read "averages"() -> (w507:i32)
        n292 = local read "ROI Top"() -> (w491:i32)
        n293 = local read "ROI Left"() -> (w489:i32)
        n294 = local read "binning"() -> (w493:u16)
        n295 = local read "ESP_t0"() -> (w480:dbl)
        n296 = Increment(x=w512) -> (x+1=w514:u16)
        n297 = Current VI's Path() -> (path=w511:path)
        n298 = local read "gain"() -> (w510:bool)
        n299 = Get Date/Time In Seconds() -> (seconds since 1Jan1904=w487:timestamp)
        n300 = call "saverunnumber.vi"("RunNumber"=w514, "VI path"=w511) -> ()  [unwired: 10 in]
        n301 = local write "RunNumber"(w514) -> ()
        n302 = call "create_opti_path.vi"("RunNumber"=w514, "base path"=w513) -> ("Path"=w484:path)  [unwired: 2 in]
        n303 = Boolean To (0,1)(Boolean=w510) -> (0, 1=w494:i16)
        n304 = Boolean To (0,1)(Boolean=w509) -> (0, 1=w488:i16)
        n305 = Build Path(base path=w484, name or relative path="info.txt") -> (appended path=w482:path)
        n306 = Format Into String(format string="ScanType=%s\\nDelayPosition=%.6f\\nTimeZero=%.6f\\nAverages=%u\\nLensMode=%s\\nVoltageRange=%s\\nKineticEnergy=%f\\nPassEnergy=%f\\nCoilCurrent=%f\\nWorkFunction=%f\\nDetectorVoltage=%f\\nScreenVoltage=%f\\nConversionVoltage=%f\\nFocusDisplacement1=%f\\nFocusDisplacement2=%f\\nExposure=%u\\nGain=%u\\nBinning=%u\\nROIbottom=%u\\nROItop=%u\\nROIright=%u\\nROIleft=%u\\nDarkImg=%u\\nStartTime=%<%Y.%m.%d %H:%M:%S>T", initial string=w482, "single" ("input 1"), w479, w480, w507, w506, w505, w504, w503, w502, w501, w500, w499, w498, w497, w496, w495, w494, w493, w492, w491, w490, w489, w488, w487) -> ()  [unwired: 1 in, 2 out]
        n307 = Build Path(base path=w484, name or relative path="AVG\\000.tsv") -> (appended path=w485:path)
        n308 = Enqueue Element(queue=w522, element="snap" ("string")) -> (error out=w516:errorcluster)  [unwired: 2 in, 2 out]
        n309 = Dequeue Element(queue=w520, error in (no error)=w516) -> (element=w515:dbl[][])  [unwired: 1 in, 3 out]
        n310 = call-poly <vilib>:"Write Delimited Spreadsheet.vi"("file path (dialog if empty)"=w485, "2D data"=w515) -> ()  [unwired: 12 in, 2 out]
      }
    }
  }
  n311 = while {
    tunnel: w10 -> [w549]
    shift-right: [w543] -> _
    shift-left: _ -> [w542]
    shift-right: [w541] -> _
    shift-left: _ -> [w539]
    shift-right: [w540] -> _
    shift-left: _ -> [w538]
    shift-right: [w535] -> _
    shift-left: 0 -> [w536]
    shift-right: [w534] -> _
    shift-left: _ -> [w533]
    shift-right: [w532] -> _
    shift-left: _ -> [w531]
    tunnel: w11 -> [w530]
    shift-right: [w529] -> _
    shift-left: _ -> [w528]
    shift-right: [w526] -> _
    shift-left: _ -> [w525]
    shift-right: [w524] -> _
    shift-left: _ -> [w523]
    i -> [w527]
    stop <- w537 stop-if-true
    # "cam"
    n312 = Preview Queue Element(queue=w549, timeout in ms (-1)=w536) -> (queue out=w548:refnum<queue>, element=w547:string)  [unwired: 1 in, 2 out]
    n313 = Match Pattern(string=w547, regular expression=":") -> (before substring=w544:string, after substring=w545:string)  [unwired: 1 in, 2 out]
    n314 = case shown="\"bench\"" w544 {
      tunnel: w548 -> [w562 w594 w624 w663 w676 _ w764 w793 w857]
      tunnel: w545 -> [_ _ _ _ _ _ _ _ _]
      tunnel: [w556 w581 w620 w662 w674 w717 w761 w782 w855] -> w543
      tunnel: w542 -> [_ _ w620 w662 w674 w717 w761 w782 w855]
      tunnel: [w561 w595 w630 u64 0 ("Hout") w673 w721 w762 w788 w854] -> w541
      tunnel: [w563 w596 w631 w659 w672 w722 w763 w776 w853] -> w540
      tunnel: w539 -> [_ w598 w634 w661 w673 w724 w766 w790 w854]
      tunnel: w538 -> [_ w597 w626 _ w672 w723 w765 w789 w853]
      tunnel: [_ _ _ _ TRUE _ _ _ _] -> w537
      tunnel: [_ _ _ _ _ _ _ _ -1] -> w535
      tunnel: [w555 w582 w625 _ _ w731 _ _ _] -> w534
      tunnel: w533 -> [w555 w582 w625 _ _ w730 _ _ _]
      tunnel: [w556 w584 w627 w657 w671 w726 w755 w791 w852] -> w532
      tunnel: w531 -> [_ w584 w627 w657 w671 w726 _ w791 w852]
      tunnel: w530 -> [_ _ _ _ _ _ _ w780 _]
      tunnel: [w553 w579 w629 w656 w669 w684 w752 w785 w851] -> w529
      tunnel: w528 -> [w553 w579 w629 w656 w669 w719 w752 w785 w851]
      tunnel: w527 -> [_ _ _ _ _ w692 _ _ _]
      tunnel: [w554 w580 w628 w655 w670 w718 w751 w784 w850] -> w526
      tunnel: w525 -> [w554 w580 w628 w655 w670 w691 w751 w784 w850]
      tunnel: [w550 w576 w614 refnum<k21> refnum ("task out") w668 w677 w750 w775 w849] -> w524
      tunnel: w523 -> [_ w576 w615 w654 w668 w677 w750 w775 w849]
      frame "init" {
        w551 = 10106 items=["Default"=-1, "RSE"=10083, "NRSE"=10078, "Differential"=10106, "Pseudodifferential"=12529] ("input terminal configuration")
        w556 = u16[][] []
        n315 = flat-sequence {
          tunnel: [w565] -> w560
          tunnel: [w566] -> w559
          tunnel: [w574] -> w561
          tunnel: [w575] -> w563
          tunnel: w560 -> [w575]
          tunnel: w559 -> [w574]
          frame #0 {
            n316 = local write "cam_con?"(FALSE ("cam_con?")) -> ()
          }
          frame #1 {
            n317 = call "SCInitBoard.vi"("boardnr"="board number") -> ("Hout"=w569:u32, "error out"=w570:errorcluster)  [unwired: 1 in, 1 out]
            n318 = call "SCSetupCamera.vi"("Handle"=w569, "error in (no error)"=w570) -> ("Hout"=w571:u64, "error out"=w572:errorcluster)  [unwired: 1 out]
            n319 = call "SCStopCOC.vi"("error in (no error)"=w572, "Stop mode"=0, "Handle"=w571) -> ("error out"=w565:errorcluster, "Hout"=w566:u64)
          }
          frame #2 {
            n320 = local write "cam_con?"(TRUE ("cam_con?")) -> ()
          }
        }
        n321 = Dequeue Element(queue=w562) -> (queue out=w558:refnum<queue>)  [unwired: 2 in, 3 out]
        n322 = Enqueue Element At Opposite End(queue=w558, element="set") -> ()  [unwired: 2 in, 3 out]
        n323 = call-poly <vilib>:"DAQmx Create Virtual Channel.vi"("input terminal configuration"=w551, "physical channels"=tag "Dev2/ai0") -> ("task out"=w550:refnum<k21>)  [unwired: 12 in, 1 out]
      }
      frame "set" {
        n324 = Dequeue Element(queue=w594) -> ()  [unwired: 2 in, 4 out]
        n325 = call "SCStopCOC.vi"("error in (no error)"=w597, "Stop mode"=0, "Handle"=w598) -> ("error out"=w613:errorcluster, "Hout"=w612:u64)
        n326 = Bundle By Name(cluster=cluster{"Delay":dbl, "Exposure ":dbl} {"Delay"=0.0, "Exposure "=0.0} ("Delay and exposure"), "Exposure"="exposure [ms]") -> (w591:cluster{"Delay":dbl, "Exposure ":dbl})
        n327 = Bundle By Name(cluster=T6 {"Camera type"=0, "Operating mode\nHP & QE / HS & DiCam Pro "=0, "Frame trigger \n(High Performance and QE only)"=0, "Sequence trigger"=0, "Low Light\n(QE only)"=FALSE, "Gain"=FALSE, "Horzontal\nbinning"=0, "Vertical\nbinning "=0, "ROI Left"=1, "ROI Right"=20, "ROI Top"=1, "ROI Bottom"=15} ("Camera controls"), "Operating mode\nHP & QE / HS & DiCam Pro"="Operating mode\nHP & QE / HS & DiCam Pro", "Horzontal\nbinning"="binning", "Vertical\nbinning"="binning", "ROI Left"="ROI Left", "ROI Right"="ROI Right", "ROI Top"="ROI Top", "ROI Bottom"="ROI Bottom", "Gain"="gain", "Frame trigger \n(High Performance and QE only)"="Frame trigger \n(High Performance and QE only)") -> (w608:T6)
        n328 = call "New delay and exposure forma.vi"("Operating mode\nHP & QE / HS & DiCam Pro"="Operating mode\nHP & QE / HS & DiCam Pro", "Delay and exposure"=w591) -> ("Output table"=w609:string)  [unwired: 3 in]
        n329 = call "SCSetCoC.vi"("error in (no error)"=w613, "Delay and exposure table"=w609, "Camera controls"=w608, "Handle"=w612) -> ("error out"=w601:errorcluster, "Hout"=w600:u64)  [unwired: 1 out]
        n330 = call "SCGetImageSize.vi"("Handle"=w600, "error in (no error)"=w601) -> ("Hout"=w599:u64, "error out"=w583:errorcluster, "Horizontal size"=w588:i32, "Vertical size"=w587:i32)  [unwired: 2 out]
        n331 = Greater?(x=w588, y=w587) -> (0:w589:bool)
        n332 = Initialize Array(u16 0 ("dimension size"), w587, w588) -> (w581:u16[][])
        n333 = call "SCRun.vi"("error in (no error)"=w583, "Run mode"=0, "Handle"=w599) -> ("error out"=w596:errorcluster, "Hout"=w595:u64)  [unwired: 1 out]
        n334 = Select(t=w588, s=w589, f=w587) -> (s? t:f=w586:i32)
        n335 = property on="mainimg" class="IntGraph (strict)"("XScale.Maximum"=w586, "YScale.Maximum"=w586) -> ()  [unwired: 2 in, 2 out]
      }
      frame "bench" {
        n336 = Dequeue Element(queue=w624) -> ()  [unwired: 2 in, 4 out]
        n337 = call "SCStopCOC.vi"("error in (no error)"=w626, "Stop mode"=0, "Handle"=w634) -> ("error out"=w618:errorcluster, "Hout"=w619:u64)
        n338 = while {
          tunnel: w620 -> [w649]
          tunnel: w619 -> [w648]
          tunnel: w618 -> [w639]
          shift-right: [w645] -> _
          shift-left: _ -> [w644]
          tunnel: [w641] -> w617
          tunnel: [w640] -> w616
          tunnel: w615 -> [w636]
          tunnel: [w635] -> w614
          stop <- "stop" stop-if-true
          n339 = call "wait4trig.vi"("error in"=w639, "task/channels in"=w636) -> ("error out"=w638:errorcluster, "voltage out"=→"voltage out":dbl, "task out"=w635:refnum<k21>)  [unwired: 7 in]
          n340 = call "SCRun.vi"("error in (no error)"=w638, "Run mode"=4, "Handle"=w648) -> ("error out"=w650:errorcluster, "Hout"=w651:u64)  [unwired: 1 out]
          n341 = call <vilib>:"High Resolution Relative Seconds.vi"() -> ("relative seconds"=w645:dbl)
          n342 = call "grabimg.vi"("array in"=w649, "error in"=w650, "Hin"=w651) -> ("error out"=w640:errorcluster, "imgdata"=→"sideimg 2":i32[][], "Hout"=w641:u64)  [unwired: 6 in]
          n343 = Subtract(x=w645, y=w644) -> (x-y=w642:dbl)
          "x/y" <- w642
          n344 = Reciprocal(x=w642) -> (1/x=→"1/x":dbl)
        }
        n345 = call "SCStopCOC.vi"("error in (no error)"=w616, "Stop mode"=0, "Handle"=w617) -> ("error out"=w621:errorcluster, "Hout"=w622:u64)
        n346 = call "SCRun.vi"("error in (no error)"=w621, "Run mode"=0, "Handle"=w622) -> ("error out"=w631:errorcluster, "Hout"=w630:u64)  [unwired: 1 out]
      }
      frame "release" {
        n347 = Dequeue Element(queue=w663) -> ()  [unwired: 2 in, 4 out]
        n348 = flat-sequence {
          tunnel: w661 -> [w665]
          tunnel: [w664] -> w658
          tunnel: [w667] -> w659
          tunnel: w658 -> [w667]
          frame #0 {
            n349 = call "SCCloseBoard.vi"("Handle"=w665) -> ("error out"=w664:errorcluster)  [unwired: 1 in, 2 out]
          }
          frame #1 {
            n350 = local write "cam_con?"(FALSE ("cam_con?")) -> ()
          }
        }
        n351 = call <vilib>:"DAQmx Clear Task.vi"("task in"=w654) -> ()  [unwired: 14 in, 1 out]
      }
      frame "close" {
        n352 = Release Queue(queue=w676) -> ()  [unwired: 2 in, 3 out]
      }
      frame "idle", Default {
        n353 = call "grabimg.vi"("array in"=w717, "error in"=w723, "Hin"=w724) -> ("error out"=w722:errorcluster, "imgdata"=w720:i32[][], "Hout"=w721:u64)  [unwired: 6 in]
        n354 = local read "lower threshold"() -> (w715:i32)
        n355 = case shown="False" "cam_dark?" {
          tunnel: w726 -> [_ w749]
          tunnel: [w746 w748] -> w716
          tunnel: w720 -> [w746 w747]
          frame False {
          }
          frame True {
            n356 = Subtract(x=w747, y=w749) -> (x-y=w748:dbl[][])
          }
        }
        n357 = call "filtr_b.vi"("threshold"=w715, "input array"=w716) -> ("output array"=w707:dbl[][])  [unwired: 9 in]
        n358 = call <vilib>:"High Resolution Relative Seconds.vi"() -> ("relative seconds"=w731:dbl)
        n359 = Subtract(x=w731, y=w730) -> (x-y=w729:dbl)
        n360 = Array Size(array=w707) -> (size(s)=w706:i32[])
        n361 = Reciprocal(x=w729) -> (1/x=→"cam_fps":dbl)
        n362 = Index Array(array=w706) -> (element #1=w701:i32, element #2=w700:i32)  [unwired: 2 in]
        n363 = Subtract(x=w692, y=w691) -> (x-y=w690:i32)
        n364 = Less Or Equal?(x="pics2avg", y=w690) -> (x <= y?=w713:bool)
        n365 = And(x="reset every n pics", y=w713) -> (x .and. y?=w711:bool)
        n366 = Not(x=w711) -> (.not. x?=w710:bool)
        n367 = call-poly <vilib>:"Ramp Pattern.vi"("start"=0.0, "end"=w701, "samples"=w701) -> ("Ramp Pattern"=w696:dbl[])  [unwired: 7 in, 1 out]
        n368 = call-poly <vilib>:"Ramp Pattern.vi"("start"=0.0, "end"=w700, "samples"=w700) -> ("Ramp Pattern"=w697:dbl[])  [unwired: 7 in, 1 out]
        n369 = property on="mainimg" class="IntGraph (strict)"() -> ("CrsrLis"=w689:T4)  [unwired: 2 in, 2 out]
        n370 = And(x="cam_liveavg", y=w710) -> (x .and. y?=w708:bool)
        n371 = case shown="False" w708 {
          tunnel: w707 -> [w736 w742]
          tunnel: [w736 w739] -> w684
          tunnel: w719 -> [_ w744]
          tunnel: w692 -> [w737 _]
          tunnel: [w737 w745] -> w718
          tunnel: w691 -> [_ w745]
          tunnel: w690 -> [_ w738]
          frame False {
          }
          frame True {
            n372 = Multiply(x=w744, y=w738) -> (x*y=w743:dbl[][])
            n373 = Increment(x=w738) -> (x+1=w740:i32)
            n374 = Add(x=w743, y=w742) -> (x+y=w741:dbl[][])
            n375 = Divide(x=w741, y=w740) -> (x/y=w739:dbl[][])
          }
        }
        "mainimg" <- w684
        n376 = Index Array(array=w689) -> (element #1=w687:T7, element #2=w688:T7)  [unwired: 2 in]
        n377 = Unbundle By Name(w687) -> ("Position.X"=w681:dbl, "Position.Y"=w683:dbl)
        n378 = Unbundle By Name(w688) -> ("Position.X"=w685:dbl, "Position.Y"=w686:dbl)
        n379 = Array Max & Min(array=w684) -> (max value=→"max":dbl)  [unwired: 3 out]
        n380 = Subtract(x=w686, y=w683) -> (x-y=w682:dbl)
        n381 = Subtract(x=w685, y=w681) -> (x-y=w680:dbl)
        n382 = Array Subset(array=w684, index (row)=w683, length (row)=w682) -> (w695:dbl[][])  [unwired: 2 in]
        n383 = Array Subset(array=w684, index (col)=w681, length (col)=w680) -> (w693:dbl[][])  [unwired: 2 in]
        n384 = Array Subset(array=w684, index (row)=w683, length (row)=w682, index (col)=w681, length (col)=w680) -> (w679:dbl[][])
        n385 = Transpose 2D Array(2D array=w695) -> (transposed array=w694:dbl[][])
        n386 = Add Array Elements(numeric array=w679) -> (sum=→"sum" →"Waveform Chart":dbl)
        n387 = for {
          tunnel: w693 -> [w733] mode=indexing
          tunnel: [w732] -> w703 mode=indexing
          n388 = Add Array Elements(numeric array=w733) -> (sum=w732:dbl)
        }
        n389 = for {
          tunnel: w694 -> [w735] mode=indexing
          tunnel: [w734] -> w702 mode=indexing
          n390 = Add Array Elements(numeric array=w735) -> (sum=w734:dbl)
        }
        n391 = Bundle("Ramp Pattern"=w697, w702) -> (→"G2 X":cluster{"Ramp Pattern":dbl[], dbl[]})  [unwired: 1 in]
        n392 = Bundle(w703, "Ramp Pattern"=w696) -> (→"G2 Y":cluster{dbl[], "Ramp Pattern":dbl[]})  [unwired: 1 in]
      }
      frame "dark" {
        n393 = Dequeue Element(queue=w764) -> ()  [unwired: 2 in, 4 out]
        n394 = Array Size(array=w761) -> (size(s)=w760:i32[])
        n395 = Index Array(array=w760) -> (element #1=w759:i32, element #2=w758:i32)  [unwired: 2 in]
        n396 = Initialize Array(0.0 ("element"), w759, w758) -> (w756:dbl[][])
        n397 = for {
          N: "dark avg" -> [_]
          tunnel: w766 -> [w774]
          tunnel: w765 -> [w773]
          tunnel: [w772] -> w763
          tunnel: w761 -> [w771]
          tunnel: [w770] -> w762
          shift-right: [w767] -> w754
          shift-left: w756 -> [w768]
          n398 = call "grabimg.vi"("array in"=w771, "error in"=w773, "Hin"=w774) -> ("error out"=w772:errorcluster, "imgdata"=w769:i32[][], "Hout"=w770:u64)  [unwired: 6 in]
          n399 = Add(x=w769, y=w768) -> (x+y=w767:dbl[][])
        }
        n400 = Divide(x=w754, y="dark avg") -> (x/y=w755:dbl[][])
      }
      frame "snap" {
        n401 = Dequeue Element(queue=w793) -> ()  [unwired: 2 in, 4 out]
        n402 = local read "cam_dark?"() -> (w792:bool)
        n403 = local read "averages"() -> (w787:i32)
        n404 = To Double Precision Float(number=w782) -> (double precision float=w781:dbl[][])
        n405 = Equal To 0?(x="aq.mode") -> (x = 0?=w778:bool)
        n406 = Get Date/Time In Seconds() -> (seconds since 1Jan1904=w783:timestamp)
        n407 = for {
          N: w787 -> [w801]
          shift-right: [w821] -> w788
          shift-left: w790 -> [w823]
          shift-right: [w808] -> w786
          shift-left: w789 -> [w822]
          tunnel: w792 -> [w819]
          tunnel: w791 -> [w818]
          tunnel: w782 -> [w817]
          tunnel: w783 -> [w813]
          tunnel: w778 -> [w803]
          shift-right: [w802] -> w777
          shift-left: w781 -> [w804]
          i -> [w798]
          stop <- "abort acq." stop-if-true
          n408 = call "grabimg.vi"("array in"=w817, "error in"=w822, "Hin"=w823) -> ("error out"=w808:errorcluster, "imgdata"=w820:i32[][], "Hout"=w821:u64)  [unwired: 6 in]
          n409 = local read "lower threshold"() -> (w796:i32)
          n410 = Increment(x=w798) -> (x+1=w799:i32)
          "acq. imgs" <- w799
          n411 = Get Date/Time In Seconds() -> (seconds since 1Jan1904=w816:timestamp)
          n412 = case shown="True" w819 {
            tunnel: w820 -> [w845 w848]
            tunnel: w818 -> [_ w847]
            tunnel: [w845 w846] -> w795
            frame False {
            }
            frame True {
              n413 = Subtract(x=w848, y=w847) -> (x-y=w846:dbl[][])
            }
          }
          n414 = Divide(x=w799, y=w801) -> (x/y=→"snap_prog":dbl)
          n415 = Subtract(x=w816, y=w813) -> (x-y=w815:dbl)
          n416 = call "filtr_b.vi"("threshold"=w796, "input array"=w795) -> ("output array"=w794:dbl[][])  [unwired: 9 in]
          n417 = Divide(x=w815, y=w798) -> (x/y=w811:dbl)
          n418 = Multiply(x=w811, y=w801) -> (x*y=w814:dbl)
          n419 = Reciprocal(x=w811) -> (1/x=w810:dbl)
          n420 = case shown="True" "count?" {
            tunnel: w794 -> [w834 w836]
            tunnel: "e-size" -> [_ w838]
            tunnel: w796 -> [_ w837]
            tunnel: [w834 w835] -> w805
            frame False {
            }
            frame True {
              n421 = Array Size(array=w836) -> (size(s)=w840:i32[])
              n422 = call "findr.vi"("thresh"=w837, "esize"=w838, "inp array"=w836) -> ("locs"=w839:i32[][])  [unwired: 8 in]
              n423 = Index Array(array=w840) -> (element #1=w842:i32, element #2=w841:i32)  [unwired: 2 in]
              n424 = call "drawe.vi"("Ysize"=w842, "Xsize"=w841, "pos array"=w839) -> ("img out"=w835:i32[][])  [unwired: 8 in]
            }
          }
          n425 = Add(x=w814, y=w813) -> (x+y=→"ETA":timestamp)
          n426 = local write "cam_fps"(w810) -> ()
          n427 = case shown="True" w803 {
            tunnel: w805 -> [w824 w832]
            tunnel: w798 -> [_ w831]
            tunnel: w804 -> [w826 w830]
            tunnel: [w825 w827] -> w802
            frame False {
              n428 = Add(x=w824, y=w826) -> (x+y=w825:dbl[][])
            }
            frame True {
              n429 = Multiply(x=w830, y=w831) -> (x*y=w833:dbl[][])
              n430 = Increment(x=w831) -> (x+1=w828:i32)
              n431 = Add(x=w832, y=w833) -> (x+y=w829:dbl[][])
              n432 = Divide(x=w829, y=w828) -> (x/y=w827:dbl[][])
            }
          }
          n433 = local write "mainimg"(w794) -> ()
          n434 = Transpose 2D Array(2D array=w794) -> (transposed array=w809:dbl[][])
          n435 = for {
            tunnel: w809 -> [w844] mode=indexing
            tunnel: [w843] -> _ mode=indexing
            n436 = Add Array Elements(numeric array=w844) -> (sum=w843:dbl)
          }
          n437 = local write "sideimg"(w802) -> ()
        }
        n438 = Enqueue Element(queue=w780, element=w777, error in (no error)=w786) -> (error out=w776:errorcluster)  [unwired: 1 in, 2 out]
      }
      frame "suspend" {
        n439 = Dequeue Element(queue=w857) -> ()  [unwired: 2 in, 4 out]
      }
    }
    "cam_error" <- w540
  }
  n440 = while {
    tunnel: w10 -> [w863]
    tunnel: w13 -> [w862]
    tunnel: w3 -> [w861]
    tunnel: w24 -> [w860]
    tunnel: w2 -> [w858]
    tunnel: w11 -> [w859]
    stop <- w864 stop-if-true
    n441 = event shown="[12] \"delscan_go 2\": Value Change" {
      selector: _ -> [_ _ _ _ _ _ _ _ _ _ _ _ _ _ _ _ _ _ _ _ _ _ _ _ _ _ _]
      dyn-events: _ -> [_ _ _ _ _ _ _ _ _ _ _ _ _ _ _ _ _ _ _ _ _ _ _ _ _ _ _]
      timeout: _ -> [_ _ _ _ _ _ _ _ _ _ _ _ _ _ _ _ _ _ _ _ _ _ _ _ _ _ _]
      tunnel: [_ TRUE _ _ _ _ _ _ _ _ _ _ _ _ _ _ _ _ _ _ _ _ _ _ _ _ _] -> w864
      tunnel: w863 -> [_ w877 w880 _ _ _ _ _ w906 w908 _ _ _ _ _ _ _ _ _ _ _ _ _ _ _ _ w1015]
      tunnel: w862 -> [_ w876 _ w884 _ _ _ _ _ _ _ _ _ _ _ _ _ w941 _ w953 _ _ _ _ _ _ _]
      tunnel: w861 -> [_ w875 _ _ w890 _ _ _ _ _ _ _ _ _ w929 _ w933 _ _ _ _ _ _ _ _ _ _]
      tunnel: w860 -> [_ w874 _ _ _ w896 w902 w903 _ _ _ _ _ _ _ _ _ _ _ _ _ _ _ _ _ _ _]
      tunnel: w859 -> [_ w868 _ _ _ _ _ _ _ _ _ _ _ _ _ _ _ _ _ _ _ _ _ _ _ _ _]
      tunnel: w858 -> [_ w867 _ _ _ _ _ _ _ _ w910 w912 w913 _ _ w931 _ _ _ _ _ _ _ _ _ w1014 _]
      event Timeout {
        n442 = event-data() -> ()  [unwired: 1 in, 1 out]
        n443 = call-poly <vilib>:"Read Delimited Spreadsheet.vi"() -> ("all rows"=w865:string[][])  [unwired: 10 in, 5 out]
        n444 = local write "delay table [fs]"(w865) -> ()
      }
      event "main_close": Value Change {
        w866 = "close" ("element")
        w873 = "release" ("element")
        n445 = event-data() -> ()  [unwired: 1 in, 1 out]
        n446 = Release Queue(queue=w868) -> ()  [unwired: 2 in, 3 out]
        n447 = Enqueue Element(queue=w877, element=w873) -> (queue out=w872:refnum<queue>)  [unwired: 2 in, 2 out]
        n448 = Enqueue Element(queue=w876, element=w873) -> (queue out=w871:refnum<queue>)  [unwired: 2 in, 2 out]
        n449 = Enqueue Element(queue=w875, element=w873) -> (queue out=w870:refnum<queue>)  [unwired: 2 in, 2 out]
        n450 = Enqueue Element(queue=w874, element=w873) -> (queue out=w869:refnum<queue>)  [unwired: 2 in, 2 out]
        n451 = Enqueue Element(queue=w872, element=w866) -> ()  [unwired: 2 in, 3 out]
        n452 = Enqueue Element(queue=w871, element=w866) -> ()  [unwired: 2 in, 3 out]
        n453 = Enqueue Element(queue=w870, element=w866) -> ()  [unwired: 2 in, 3 out]
        n454 = Enqueue Element(queue=w869, element=w866) -> ()  [unwired: 2 in, 3 out]
        n455 = Enqueue Element(queue=w867, element=w866) -> ()  [unwired: 2 in, 3 out]
      }
      event "cam_release", "cam_init": Value Change {
        n456 = event-data() -> ()  [unwired: 1 in, 2 out]
        n457 = Select(t="init" ("name (unnamed)"), s="cam_init", f="release" ("name (unnamed)")) -> (s? t:f=w879:string)
        n458 = Enqueue Element(queue=w880, element=w879) -> ()  [unwired: 2 in, 3 out]
      }
      event "ESP_release", "ESP_init": Value Change {
        n459 = event-data() -> ()  [unwired: 1 in, 2 out]
        n460 = Select(t="init" ("name (unnamed)"), s="ESP_init", f="release" ("name (unnamed)")) -> (s? t:f=w888:string)
        n461 = Enqueue Element(queue=w884, element=w888) -> ()  [unwired: 2 in, 3 out]
      }
      event "manip_init", "manip_release": Value Change {
        n462 = event-data() -> ()  [unwired: 1 in, 2 out]
        n463 = Flush Queue(queue=w890) -> (queue out=w889:refnum<queue>)  [unwired: 1 in, 2 out]
        n464 = Select(t="init" ("name (unnamed)"), s="manip_init", f="release" ("name (unnamed)")) -> (s? t:f=w892:string)
        n465 = Enqueue Element(queue=w889, element=w892) -> ()  [unwired: 2 in, 3 out]
      }
      event "phoib_release", "phoib_init": Value Change {
        n466 = event-data() -> ()  [unwired: 1 in, 2 out]
        n467 = Flush Queue(queue=w896) -> (queue out=w895:refnum<queue>)  [unwired: 1 in, 2 out]
        n468 = Select(t="init" ("name (unnamed)"), s="phoib_init", f="release" ("name (unnamed)")) -> (s? t:f=w898:string)
        n469 = Enqueue Element(queue=w895, element=w898) -> ()  [unwired: 2 in, 3 out]
      }
      event "phoib_standby": Value Change {
        n470 = event-data() -> ()  [unwired: 1 in, 2 out]
        n471 = Enqueue Element(queue=w902, element="standby") -> ()  [unwired: 2 in, 3 out]
      }
      event "phoib_set": Value Change {
        n472 = event-data() -> ()  [unwired: 1 in, 2 out]
        n473 = Enqueue Element(queue=w903, element="set") -> ()  [unwired: 2 in, 3 out]
      }
      event "cam_dark": Value Change {
        n474 = event-data() -> ()  [unwired: 1 in, 2 out]
        n475 = Enqueue Element(queue=w906, element="dark") -> ()  [unwired: 2 in, 3 out]
      }
      event "ROI Left", "ROI Right", "ROI Top", "ROI Bottom", "exposure [ms]", "binning", "gain": Value Change {
        n476 = event-data() -> ()  [unwired: 1 in, 1 out]
        n477 = Enqueue Element(queue=w908, element="set") -> ()  [unwired: 2 in, 3 out]
      }
      event "cam_saveimg": Value Change {
        n478 = event-data() -> ()  [unwired: 1 in, 1 out]
        n479 = Enqueue Element(queue=w910, element="single") -> ()  [unwired: 2 in, 3 out]
      }
      event "delscan_go": Value Change {
        n480 = event-data() -> ()  [unwired: 1 in, 1 out]
        n481 = Enqueue Element(queue=w912, element="GO") -> ()  [unwired: 2 in, 3 out]
      }
      event "delscan_go 2": Value Change {
        n482 = event-data() -> ()  [unwired: 1 in, 1 out]
        n483 = Enqueue Element(queue=w913, element="delscan_chop") -> ()  [unwired: 2 in, 3 out]
      }
      event "Move Abs": Value Change {
        n484 = event-data() -> ()  [unwired: 1 in, 1 out]
      }
      event "ManipRel +", "ManipRel -": Value Change {
        n485 = event-data() -> ()  [unwired: 1 in, 2 out]
        n486 = Negate(x="manip_deltas") -> (-x=w917:dbl[])
        n487 = Select(t="manip_deltas", s="ManipRel +", f=w917) -> (s? t:f=w915:dbl[])
        n488 = Index Array(array=w915) -> (element #1=w921:dbl, element #2=w922:dbl, element #3=w923:dbl, element #4=w924:dbl, element #5=w925:dbl, element #6=w926:dbl)  [unwired: 6 in]
        n489 = Format Into String(format string="%g_%g_%g_%g_%g_%g", w921, w922, w923, w924, w925, w926) -> (resulting string=w928:string)  [unwired: 2 in, 1 out]
        n490 = Concatenate Strings("relative:" ("string"), w928) -> (w919:string)
        n491 = Enqueue Element(queue=w929, element=w919) -> ()  [unwired: 2 in, 3 out]
      }
      event "Optimize": Value Change {
        n492 = event-data() -> ()  [unwired: 1 in, 6 out]
        n493 = Enqueue Element(queue=w931, element="manip") -> ()  [unwired: 2 in, 3 out]
      }
      event "stop manip": Value Change {
        n494 = event-data() -> ()  [unwired: 1 in, 1 out]
        n495 = Enqueue Element(queue=w933, element="stop") -> ()  [unwired: 2 in, 3 out]
      }
      event "ESP_go": Value Change {
        w935 = ":" ("string")
        n496 = event-data() -> ()  [unwired: 1 in, 1 out]
        n497 = local read "ESP Axis"() -> (w934:i32)
        n498 = Number To Decimal String(number=w934) -> (decimal integer string=w937:string)  [unwired: 1 in]
        n499 = Number To Fractional String(number="ESP_dest") -> (F-format string=w936:string)  [unwired: 3 in]
        n500 = Concatenate Strings("abs:" ("string"), w937, w935, w936, w935) -> (w940:string)
        n501 = Enqueue Element(queue=w941, element=w940) -> ()  [unwired: 2 in, 3 out]
      }
      event "ESP_set_t0": Value Change {
        n502 = event-data() -> ()  [unwired: 1 in, 1 out]
        n503 = Current VI's Path() -> (path=w947:path)
        n504 = Strip Path(path=w947) -> (stripped path=w943:path)  [unwired: 1 out]
        n505 = Strip Path(path=w943) -> (stripped path=w942:path)  [unwired: 1 out]
        n506 = local read "ESP_pos"() -> (w945:dbl)
        "ESP_t0" <- w945
        n507 = Number To Fractional String(number=w945) -> (F-format string=w944:string)  [unwired: 3 in]
        n508 = Build Path(base path=w942, name or relative path="t0.txt") -> (appended path=w946:path)
        n509 = Write to Text File(file (use dialog)=w946, text=w944) -> ()  [unwired: 2 in, 3 out]
      }
      event "ESP_+", "ESP_-": Value Change {
        n510 = event-data() -> ()  [unwired: 1 in, 6 out]
        n511 = Negate(x="ESP_delta") -> (-x=w956:dbl)
        n512 = Select(t="ESP_delta", s="ESP_+", f=w956) -> (s? t:f=w954:dbl)
        n513 = Number To Decimal String(number="ESP Axis") -> (decimal integer string=w951:string)  [unwired: 1 in]
        n514 = Number To Fractional String(number=w954) -> (F-format string=w949:string)  [unwired: 3 in]
        n515 = Concatenate Strings("rel:" ("string"), w951, ":" ("string"), w949) -> (w959:string)
        n516 = Enqueue Element(queue=w953, element=w959) -> ()  [unwired: 2 in, 3 out]
      }
      event "ESP_dest": Value Change {
        n517 = event-data() -> ()  [unwired: 1 in, 6 out]
        n518 = local read "ESP_dest"() -> (w963:dbl)
        n519 = local read "ESP_t0"() -> (w962:dbl)
        n520 = call "mm2time.vi"("fs?"=TRUE ("fs[1]/ps[0]"), "Offset (mm)"=w962, "distance (mm)"=w963) -> ("time in fs/ps seconds"=w960:dbl)
        n521 = local write "ESP_dest_t"(w960) -> ()
      }
      event "ESP_dest_t": Value Change {
        n522 = event-data() -> ()  [unwired: 1 in, 1 out]
        n523 = local read "ESP_t0"() -> (w966:dbl)
        n524 = call "time2mm.vi"("fs[1]/ps[0]"=TRUE, "Offset (mm)"=w966, "time"="ESP_dest_t") -> ("position (mm)"=w964:dbl)
        n525 = local write "ESP_dest"(w964) -> ()
      }
      event "load delay table": Value Change {
        n526 = event-data() -> ()  [unwired: 1 in, 6 out]
        n527 = call-poly <vilib>:"Read Delimited Spreadsheet.vi"() -> ("all rows"=w969:string[][])  [unwired: 10 in, 5 out]
        n528 = local read "binning"() -> (w976:u16)
        n529 = local write "delay table [fs]"(w969) -> ()
        n530 = local read "delscan_iters"() -> (w970:u32)
        n531 = local read "time / step"() -> (w979:dbl)
        n532 = Array Size(array=w969) -> (size(s)=w980:i32[])
        n533 = Index Array(array=dbl[] [8.79, 2.2, 0.553, 0.138], index=w976) -> (element=w974:dbl)
        n534 = Index Array(array=w980) -> (element #1=w968:i32)  [unwired: 2 in, 1 out]
        n535 = Multiply(x=w970, y=w968) -> (x*y=w973:u32)
        n536 = Multiply(x=w968, y=w974) -> (x*y=w975:dbl)
        n537 = Multiply(x=w973, y=w979) -> (x*y=w978:dbl)
        n538 = Increment(x=w973) -> (x+1=w972:u32)
        n539 = Multiply(x=w972, y=w974) -> (x*y=w971:dbl)
        n540 = local write "delaypoints"(w968) -> ()
        n541 = local write "total steps"(w973) -> ()
        n542 = local write "duration [HH:MM:SS]"(w978) -> ()
        n543 = local write "RAM [MB]"(w975) -> ()
        n544 = local write "disk [MB]"(w971) -> ()
      }
      event "delay table [fs]", "delscan_iters": Value Change {
        n545 = event-data() -> ()  [unwired: 1 in, 6 out]
        n546 = local read "binning"() -> (w989:u16)
        n547 = local read "delay table [fs]"() -> (w993:string[][])
        n548 = local read "delscan_iters"() -> (w983:u32)
        n549 = local read "time / step"() -> (w991:dbl)
        n550 = Array Size(array=w993) -> (size(s)=w992:i32[])
        n551 = Index Array(array=dbl[] [8.79, 2.2, 0.553, 0.138], index=w989) -> (element=w987:dbl)
        n552 = Index Array(array=w992) -> (element #1=w981:i32)  [unwired: 2 in, 1 out]
        n553 = Multiply(x=w983, y=w981) -> (x*y=w986:u32)
        n554 = Multiply(x=w981, y=w987) -> (x*y=w988:dbl)
        n555 = Multiply(x=w986, y=w991) -> (x*y=w990:dbl)
        n556 = Increment(x=w986) -> (x+1=w985:u32)
        n557 = Multiply(x=w985, y=w987) -> (x*y=w984:dbl)
        n558 = local write "delaypoints"(w981) -> ()
        n559 = local write "total steps"(w986) -> ()
        n560 = local write "duration [HH:MM:SS]"(w990) -> ()
        n561 = local write "RAM [MB]"(w988) -> ()
        n562 = local write "disk [MB]"(w984) -> ()
      }
      event "generate delay table": Value Change {
        n563 = event-data() -> ()  [unwired: 1 in, 1 out]
        n564 = call "getdelaypoints.vi"("delscan_stepsize"="delscan_stepsize", "delscan_end"="delscan_end", "delscan_start"="delscan_start") -> ("delaypoints"=w1009:dbl[])
        n565 = Number To Fractional String(number=w1009) -> (F-format string=w1008:string[])  [unwired: 3 in]
        n566 = Build Array(w1008) -> (w1007:string[][])
        n567 = Transpose 2D Array(2D array=w1007) -> (transposed array=w994:string[][])
        n568 = local write "delay table [fs]"(w994) -> ()
        n569 = local read "binning"() -> (w1003:u16)
        n570 = local read "delscan_iters"() -> (w997:u32)
        n571 = local read "time / step"() -> (w1005:dbl)
        n572 = Array Size(array=w994) -> (size(s)=w1006:i32[])
        n573 = Index Array(array=dbl[] [8.79, 2.2, 0.553, 0.138], index=w1003) -> (element=w1001:dbl)
        n574 = Index Array(array=w1006) -> (element #1=w995:i32)  [unwired: 2 in, 1 out]
        n575 = Multiply(x=w997, y=w995) -> (x*y=w1000:u32)
        n576 = Multiply(x=w995, y=w1001) -> (x*y=w1002:dbl)
        n577 = Multiply(x=w1000, y=w1005) -> (x*y=w1004:dbl)
        n578 = Increment(x=w1000) -> (x+1=w999:u32)
        n579 = Multiply(x=w999, y=w1001) -> (x*y=w998:dbl)
        n580 = local write "delaypoints"(w995) -> ()
        n581 = local write "total steps"(w1000) -> ()
        n582 = local write "duration [HH:MM:SS]"(w1004) -> ()
        n583 = local write "RAM [MB]"(w1002) -> ()
        n584 = local write "disk [MB]"(w998) -> ()
      }
      event "mainimg": Cursor Release {
        n585 = event-data() -> ()  [unwired: 1 in, 1 out]
        n586 = Enqueue Element(queue=w1014, element="refresh") -> ()  [unwired: 2 in, 3 out]
      }
      event "dev_bench": Value Change {
        n587 = event-data() -> ()  [unwired: 1 in, 2 out]
        n588 = Enqueue Element(queue=w1015, element="bench") -> ()  [unwired: 2 in, 3 out]
      }
    }
  }
  n589 = while {
    tunnel: w13 -> [w1025]
    shift-right: [w1023] -> _
    shift-left: _ -> [w1021]
    shift-right: [w1022] -> _
    shift-left: _ -> [w1020]
    shift-right: [w1018] -> _
    shift-left: 0 -> [w1019]
    tunnel: w2 -> [w1017]
    stop <- w1024 stop-if-true
    # "ESP"
    n590 = Preview Queue Element(queue=w1025, timeout in ms (-1)=w1019) -> (queue out=w1028:refnum<queue>, element=w1029:string)  [unwired: 1 in, 2 out]
    n591 = Match Pattern(string=w1029, regular expression=":") -> (before substring=w1027:string, after substring=w1026:string)  [unwired: 1 in, 2 out]
    n592 = case shown="\"idle\", Default" w1027 {
      tunnel: w1028 -> [_ w1040 w1058 w1092 w1093 w1100 w1105]
      tunnel: w1026 -> [_ w1045 w1065 _ _ _ _]
      tunnel: [_ _ _ _ _ TRUE _] -> w1024
      tunnel: [w1032 w1047 w1059 w1090 refnum<visa-resource-name> refnum ("VISA resource name out") w1097 w1104] -> w1023
      tunnel: [w1031 w1048 w1057 w1089 w1095 w1098 w1103] -> w1022
      tunnel: w1021 -> [w1036 w1050 w1063 w1090 w1096 w1097 _]
      tunnel: w1020 -> [w1035 w1049 w1064 w1089 _ w1098 _]
      tunnel: [_ _ _ -1 _ _ _] -> w1018
      tunnel: w1017 -> [_ _ w1056 _ _ _ _]
      frame "idle", Default {
        n593 = local read "ESP Axis"() -> (w1033:i32)
        n594 = local read "ESP_t0"() -> (w1039:dbl)
        n595 = call "Read Actual Position.vi"("error in (no error)"=w1035, "Axis (1)"=w1033, "VISA resource name"=w1036) -> ("error out"=w1031:errorcluster, "Position (units)"=w1034:dbl, "VISA resource name out"=w1032:refnum<visa-resource-name>)  [unwired: 2 in]
        "ESP_pos" <- w1034
        n596 = call "mm2time.vi"("fs?"=TRUE, "Offset (mm)"=w1039, "distance (mm)"=w1034) -> ("time in fs/ps seconds"=→"ESP_delay":dbl)
      }
      frame "rel" {
        n597 = Match Pattern(string=w1045, regular expression=":") -> (before substring=w1044:string, after substring=w1043:string)  [unwired: 1 in, 2 out]
        n598 = Dequeue Element(queue=w1040) -> ()  [unwired: 2 in, 4 out]
        n599 = Decimal String To Number(string=w1044) -> (number=w1042:i32)  [unwired: 2 in, 1 out]
        n600 = Fract/Exp String To Number(string=w1043) -> (number=w1041:dbl)  [unwired: 3 in, 1 out]
        n601 = call "Move Relative.vi"("error in (no error)"=w1049, "Position (0 units)"=w1041, "Axis (1)"=w1042, "VISA resource name"=w1050) -> ("error out"=w1048:errorcluster, "VISA resource name out"=w1047:refnum<visa-resource-name>)  [unwired: 2 in]
      }
      frame "abs" {
        n602 = Dequeue Element(queue=w1058) -> ()  [unwired: 2 in, 4 out]
        n603 = Match Pattern(string=w1065, regular expression=":") -> (before substring=w1066:string, after substring=w1054:string)  [unwired: 1 in, 2 out]
        n604 = Match Pattern(string=w1054, regular expression=":") -> (before substring=w1053:string, after substring=w1052:string)  [unwired: 1 in, 2 out]
        n605 = Decimal String To Number(string=w1066) -> (number=w1062:i32)  [unwired: 2 in, 1 out]
        n606 = Fract/Exp String To Number(string=w1053) -> (number=w1051:dbl)  [unwired: 3 in, 1 out]
        n607 = call "Move Absolute.vi"("error in (no error)"=w1064, "Position (0 units)"=w1051, "Axis (1)"=w1062, "VISA resource name"=w1063) -> ("error out"=w1060:errorcluster, "VISA resource name out"=w1061:refnum<visa-resource-name>)  [unwired: 2 in]
        n608 = case shown="\"wait\"" w1052 {
          tunnel: w1062 -> [_ w1074]
          tunnel: w1061 -> [w1069 w1079]
          tunnel: w1060 -> [w1068 w1078]
          tunnel: [w1069 w1071] -> w1059
          tunnel: [w1068 w1077] -> w1057
          tunnel: w1056 -> [_ w1076]
          frame "", Default {
          }
          frame "wait" {
            n609 = while {
              tunnel: w1074 -> [w1088]
              shift-right: [w1085] -> w1073
              shift-left: w1079 -> [w1087]
              shift-right: [w1084] -> w1072
              shift-left: w1078 -> [w1086]
              stop <- w1083 stop-if-true
              n610 = call "Get Axis Motion Status.vi"("error in (no error)"=w1086, "Axis (1)"=w1088, "VISA resource name"=w1087) -> ("error out"=w1084:errorcluster, "Motion Done"=w1083:bool, "VISA resource name out"=w1085:refnum<visa-resource-name>)  [unwired: 2 in]
            }
            n611 = flat-sequence {
              tunnel: w1073 -> [w1082]
              tunnel: w1072 -> [w1081]
              tunnel: [w1082] -> w1071
              tunnel: [w1081] -> w1070
              frame #0 {
                n612 = Wait (ms)(milliseconds to wait=u32 1000) -> ()  [unwired: 1 out]
              }
            }
            n613 = Enqueue Element(queue=w1076, element="done", error in (no error)=w1070) -> (error out=w1077:errorcluster)  [unwired: 1 in, 2 out]
          }
        }
      }
      frame "suspend" {
        n614 = Dequeue Element(queue=w1092) -> ()  [unwired: 2 in, 4 out]
      }
      frame "release" {
        n615 = Dequeue Element(queue=w1093) -> ()  [unwired: 2 in, 4 out]
        n616 = call "Close.vi"("VISA resource name"=w1096) -> ("error out"=w1095:errorcluster)  [unwired: 10 in]
      }
      frame "close" {
        n617 = Release Queue(queue=w1100) -> ()  [unwired: 2 in, 3 out]
      }
      frame "init" {
        n618 = Dequeue Element(queue=w1105) -> ()  [unwired: 2 in, 4 out]
        n619 = flat-sequence {
          tunnel: [w1108] -> w1102
          tunnel: [w1107] -> w1101
          tunnel: [w1112] -> w1103
          tunnel: [w1113] -> w1104
          tunnel: w1102 -> [w1113]
          tunnel: w1101 -> [w1112]
          frame #0 {
            n620 = local write "ESP_con?"(FALSE ("ESP_con?")) -> ()
          }
          frame #1 {
            n621 = call "Initialize.vi"("VISA resource name"="ESP301 VISA", "Serial Link (RS232)"=enum16{"RS232", "USB"}."USB") -> ("VISA resource name out"=w1108:refnum<visa-resource-name>, "error out"=w1107:errorcluster)  [unwired: 7 in]
          }
          frame #2 {
            n622 = local write "ESP_con?"(TRUE ("ESP_con?")) -> ()
          }
        }
      }
    }
    "error out" <- w1022
  }
  n623 = while {
    tunnel: w3 -> [w1122]
    shift-right: [w1120] -> _
    shift-left: _ -> [w1118]
    shift-right: [w1119] -> _
    shift-left: _ -> [w1117]
    shift-right: [w1115] -> _
    shift-left: 0 -> [w1116]
    tunnel: w2 -> [w1114]
    stop <- w1121 stop-if-true
    # "manip"
    n624 = Preview Queue Element(queue=w1122, timeout in ms (-1)=w1116) -> (queue out=w1125:refnum<queue>, element=w1126:string)  [unwired: 1 in, 2 out]
    n625 = Match Pattern(string=w1126, regular expression=":") -> (before substring=w1124:string, after substring=w1123:string)  [unwired: 1 in, 2 out]
    n626 = case shown="\"init\"" w1124 {
      tunnel: w1125 -> [_ w1138 w1165 w1192 w1196 w1205 w1210]
      tunnel: w1123 -> [_ _ w1152 _ _ _ _]
      tunnel: [_ _ _ _ _ TRUE _] -> w1121
      tunnel: [w1132 w1140 w1144 w1194 refnum<k5> refnum ("gateway_connection out") w1203 w1209] -> w1120
      tunnel: [w1131 w1139 w1146 w1193 w1198 w1202 w1208] -> w1119
      tunnel: w1118 -> [w1134 w1142 w1168 w1194 w1200 w1203 _]
      tunnel: w1117 -> [w1133 w1141 w1167 w1193 _ w1202 _]
      tunnel: [_ _ _ -1 _ _ _] -> w1115
      tunnel: w1114 -> [_ _ w1143 _ _ _ _]
      frame "idle", Default {
        n627 = call "sp_manip_get_axis_status.vi"("error in"=w1133, "gateway_connection"=w1134) -> ("error out"=w1131:errorcluster, "axis_out"=w1130:T8, "gateway_connection out"=w1132:refnum<k5>)  [unwired: 5 in, 2 out]
        n628 = for {
          tunnel: w1130 -> [w1137] mode=indexing
          tunnel: [w1136] -> w1129 mode=indexing
          tunnel: [w1135] -> w1128 mode=indexing
          n629 = Unbundle By Name(w1137) -> ("Axis_Position"=w1136:dbl, "moving"=w1135:bool)
        }
        "moving?" <- w1128
        n630 = local write "pos"(w1129) -> ()
      }
      frame "stop" {
        n631 = Dequeue Element(queue=w1138) -> ()  [unwired: 2 in, 4 out]
        n632 = call "sp_manip_abort.vi"("error in"=w1141, "gateway_connection"=w1142) -> ("error out"=w1139:errorcluster, "gateway_connection out"=w1140:refnum<k5>)  [unwired: 6 in, 2 out]
      }
      frame "relative" {
        n633 = Dequeue Element(queue=w1165) -> ()  [unwired: 2 in, 4 out]
        n634 = Match Pattern(string=w1152, regular expression=":") -> (before substring=w1151:string, after substring=w1150:string)  [unwired: 1 in, 2 out]
        n635 = Equal?(x=w1150, y="wait") -> (x = y?=w1148:bool)
        n636 = call "sp_manip_get_axis_status.vi"("error in"=w1167, "gateway_connection"=w1168) -> ("error out"=w1170:errorcluster, "axis_out"=w1157:T8, "gateway_connection out"=w1169:refnum<k5>)  [unwired: 5 in, 2 out]
        n637 = Scan From String(format string="%g_%g_%g_%g_%g_%g", input string=w1151) -> (output 1=w1164:dbl, output 2=w1163:dbl, output 3=w1162:dbl, output 4=w1161:dbl, output 5=w1160:dbl, output 6=w1159:dbl)  [unwired: 8 in, 3 out]
        n638 = for {
          tunnel: w1157 -> [w1191] mode=indexing
          tunnel: [w1190] -> w1155 mode=indexing
          tunnel: [w1189] -> w1156 mode=indexing
          n639 = Unbundle By Name(w1191) -> ("Axis_Name"=w1190:string, "Axis_Position"=w1189:dbl)
        }
        n640 = Build Array(w1164, w1163, w1162, w1161, w1160, w1159) -> (w1158:dbl[])
        n641 = Add(x=w1156, y=w1158) -> (x+y=w1154:dbl[])
        n642 = call "sp_manip_start_move.vi"("error in"=w1170, "target positions"=w1154, "axis names"=w1155, "gateway_connection"=w1169) -> ("error out"=w1147:errorcluster, "gateway_connection out"=w1145:refnum<k5>)  [unwired: 4 in, 2 out]
        n643 = case shown="True" w1148 {
          tunnel: w1147 -> [w1171 w1178]
          tunnel: [w1171 w1174] -> w1146
          tunnel: w1145 -> [w1172 w1179]
          tunnel: [w1172 w1177] -> w1144
          tunnel: w1143 -> [_ w1173]
          frame False {
          }
          frame True {
            n644 = while {
              tunnel: w1179 -> [w1183]
              tunnel: w1178 -> [w1182]
              tunnel: [w1181] -> w1177
              tunnel: [w1180] -> w1175
              stop <- w1184 continue-if-true
              n645 = call "sp_manip_get_axis_status.vi"("error in"=w1182, "gateway_connection"=w1183) -> ("error out"=w1180:errorcluster, "axis_out"=w1186:T8, "gateway_connection out"=w1181:refnum<k5>)  [unwired: 5 in, 2 out]
              n646 = for {
                tunnel: w1186 -> [w1188] mode=indexing
                tunnel: [w1187] -> w1185 mode=indexing
                n647 = Unbundle By Name(w1188) -> ("moving"=w1187:bool)
              }
              n648 = Or Array Elements(Boolean array=w1185) -> (logical OR=w1184:bool)
            }
            n649 = Enqueue Element(queue=w1173, element="done", error in (no error)=w1175) -> (error out=w1174:errorcluster)  [unwired: 1 in, 2 out]
          }
        }
      }
      frame "suspend" {
        n650 = Dequeue Element(queue=w1192) -> ()  [unwired: 2 in, 4 out]
      }
      frame "release" {
        n651 = Dequeue Element(queue=w1196) -> ()  [unwired: 2 in, 4 out]
        n652 = call "sp_manip_disconnect.vi"("gateway_connection"=w1200) -> ("error out"=w1199:errorcluster, "gateway_connection_out"=w1201:refnum<k5>)  [unwired: 7 in, 2 out]
        n653 = call "tcp_gateway_close_connection.vi"("error in"=w1199, "server_connection"=w1201) -> ("error out"=w1198:errorcluster)  [unwired: 5 in]
      }
      frame "close" {
        n654 = Release Queue(queue=w1205) -> ()  [unwired: 2 in, 3 out]
      }
      frame "init" {
        n655 = Dequeue Element(queue=w1210) -> ()  [unwired: 2 in, 4 out]
        n656 = flat-sequence {
          tunnel: [w1213] -> w1207
          tunnel: [w1212] -> w1206
          tunnel: [w1223] -> w1208
          tunnel: [w1224] -> w1209
          tunnel: w1207 -> [w1224]
          tunnel: w1206 -> [w1223]
          frame #0 {
            n657 = local write "manip_con?"(FALSE ("manip_con?")) -> ()
          }
          frame #1 {
            n658 = call "tcp_gateway_open_connection.vi"() -> ("gateway_connection"=w1216:refnum<k5>, "error out"=w1215:errorcluster)  [unwired: 5 in, 3 out]
            n659 = call "sp_manip_connect.vi"("error in"=w1215, "gateway_connection"=w1216) -> ("error out"=w1212:errorcluster, "axis_out"=w1214:T8, "gateway_connection out"=w1213:refnum<k5>)  [unwired: 5 in, 2 out]
            n660 = for {
              tunnel: w1214 -> [w1221] mode=indexing
              tunnel: [w1220] -> w1217 mode=indexing
              tunnel: [w1219] -> w1218 mode=indexing
              n661 = Unbundle By Name(w1221) -> ("Axis_Name"=w1220:string, "Axis_Position"=w1219:dbl)
            }
            "axis" <- w1217
            "pos" <- w1218
            n662 = local write "dest"(w1218) -> ()
          }
          frame #2 {
            n663 = local write "manip_con?"(TRUE ("manip_con?")) -> ()
          }
        }
      }
    }
    "error out 2" <- w1119
  }
  n664 = while {
    tunnel: w24 -> [w1235]
    shift-right: [w1232] -> _
    shift-left: 0 -> [w1233]
    shift-right: [w1231] -> _
    shift-left: _ -> [w1230]
    shift-right: [w1229] -> _
    shift-left: _ -> [w1228]
    shift-right: [w1227] -> _
    shift-left: u32 0 ("pHandle") -> [w1226]
    tunnel: string[] ["Kinetic Energy", "Pass Energy", "Coil Current", "Work Function", "Detector Voltage", "Screen Voltage", "Conversion Voltage", "Focus Displacement 1", "Focus Displacement 2"] -> [w1225]
    stop <- w1234 stop-if-true
    # "phoib"
    n665 = Preview Queue Element(queue=w1235, timeout in ms (-1)=w1233) -> (queue out=w1238:refnum<queue>, element=w1239:string)  [unwired: 1 in, 2 out]
    n666 = Match Pattern(string=w1239, regular expression=":") -> (before substring=w1237:string, after substring=w1236:string)  [unwired: 1 in, 2 out]
    n667 = case shown="\"standby\"" w1237 {
      tunnel: w1238 -> [_ w1292 w1308 w1324 w1338 w1342 w1348]
      tunnel: w1236 -> [_ _ _ _ _ _ _]
      tunnel: [_ _ _ _ TRUE _ _] -> w1234
      tunnel: [_ _ _ _ _ -1 _] -> w1232
      tunnel: [w1249 w1294 w1311 w1322 w1336 w1341 w1345] -> w1231
      tunnel: w1230 -> [w1260 w1283 w1313 w1323 w1336 w1341 _]
      tunnel: [w1248 w1293 w1310 w1321 w1334 w1339 w1344] -> w1229
      tunnel: w1228 -> [w1258 w1282 w1312 _ w1334 w1339 _]
      tunnel: [w1246 w1280 w1309 w1320 w1335 w1340 w1347] -> w1227
      tunnel: w1226 -> [w1246 w1280 w1309 w1319 w1335 w1340 _]
      tunnel: w1225 -> [w1247 w1273 _ _ _ _ _]
      frame "idle", Default {
        n668 = call "SL2_AD_DLL_Phoibos_GetDeviceState.vi"("dll_path"=w1260, "pHandle_in"=w1246, "dev_type"=DEF_dev_type."devA (analyzer)", "error in"=w1258) -> ("path out"=w1245:path, "state"=→"state":T3, "error out"=w1244:errorcluster)  [unwired: 2 in]
        n669 = for {
          tunnel: w1246 -> [w1267]
          tunnel: w1247 -> [w1265] mode=indexing
          tunnel: [w1264] -> w1257 mode=indexing
          tunnel: [w1263] -> w1249
          shift-right: [w1262] -> w1248
          shift-left: w1244 -> [w1266]
          tunnel: w1245 -> [w1261]
          n670 = call "SL2_AD_DLL_Phoibos_GetVoltage.vi"("error in"=w1266, "voltage_name"=w1265, "pHandle"=w1267, "dll path in"=w1261) -> ("error out"=w1262:errorcluster, "value"=w1264:dbl, "dll path out"=w1263:path)  [unwired: 3 in]
        }
        n671 = Index Array(array=w1257) -> (element #1=→"phoib_I_1":dbl, element #2=→"phoib_I_2":dbl, element #3=→"phoib_I_3":dbl, element #4=→"phoib_I_4":dbl, element #5=→"phoib_I_5":dbl, element #6=→"phoib_I_6":dbl, element #7=→"phoib_I_7":dbl, element #8=→"phoib_I_8":dbl, element #9=→"phoib_I_9":dbl)  [unwired: 9 in]
      }
      frame "set" {
        n672 = Dequeue Element(queue=w1292) -> ()  [unwired: 2 in, 4 out]
        n673 = Multiply(x="VoltageRange", y=13) -> (x*y=w1289:i32)
        n674 = Add(x="Mode", y=w1289) -> (x+y=w1286:i32)
        n675 = Index Array(array=u32[] [251749632, 251749633, 251749634, 251749635, 251749636, 251749637, 251749638, 251749639, 251749640, 251749641, 251749642, 251749643, 251749644, 251749645, 251749646, 251749647, 251749648, 251749649, 251749650, 251749651, 251749652, 251749653, 251749654, 251749655, 251749656, 251749657, 251749658, 251749659, 251749660, 251749661, 251749662, 251749663, 251749664, 251749665, 251749666, 251749667, 251749668, 251749669, 251749670, 251749671, 251749672, 251749673, 251749674, 251749675, 251749676, 251749677, 251749678, 251749679, 251749680, 251749681, 251749682, 251749683, 251749684, 251749685, 251749686, 251749687, 251749688, 251749689, 251749690, 251749691, 251749692, 251749693, 251749694, 251749695, 251749696] ("modeIDs"), index=w1286) -> (element=w1284:u32)
        n676 = Build Array("phoib_I_1s", "phoib_I_2s", "phoib_I_3s", "phoib_I_4s", "phoib_I_5s", "phoib_I_6s", "phoib_I_7s", "phoib_I_8s", "phoib_I_9s") -> (w1272:dbl[])
        n677 = call "SL2_AD_DLL_Phoibos_SetDeviceMode.vi"("pHandle"=w1280, "error in"=w1282, "value"=w1284, "dev_type"=DEF_dev_type."devA (analyzer)", "dll path in"=w1283) -> ("error out"=w1271:errorcluster, "dll path out"=w1281:path)  [unwired: 4 in]
        n678 = for {
          tunnel: w1280 -> [w1300]
          shift-right: [w1307] -> w1294
          shift-left: w1281 -> [w1304]
          tunnel: w1273 -> [w1299] mode=indexing
          tunnel: w1272 -> [w1298] mode=indexing
          shift-right: [w1306] -> w1293
          shift-left: w1271 -> [w1302]
          n679 = call "SL2_AD_DLL_Phoibos_GetVoltageRange.vi"("error in"=w1302, "voltage_name"=w1299, "pHandle"=w1300, "dll path in"=w1304) -> ("error out"=w1301:errorcluster, "min"=w1296:dbl, "max"=w1297:dbl, "dll path out"=w1303:path)  [unwired: 2 in]
          n680 = In Range and Coerce(upper limit=w1297, x=w1298, lower limit=w1296) -> (coerced(x)=w1295:dbl)  [unwired: 1 out]
          n681 = call "SL2_AD_DLL_Phoibos_SetVoltage.vi"("commit"=TRUE, "pHandle"=w1300, "error in"=w1301, "value"=w1295, "voltageName"=w1299, "dll path in"=w1303) -> ("error out"=w1306:errorcluster, "dll path out"=w1307:path)  [unwired: 3 in]
        }
      }
      frame "standby" {
        w1314 = T3 0 items=["Off"=-1, "Standby"=0, "On"=1] ("state")
        n682 = Dequeue Element(queue=w1308) -> ()  [unwired: 2 in, 4 out]
        n683 = call "SL2_AD_DLL_Phoibos_SetDeviceState.vi"("pHandle_in"=w1309, "error in"=w1312, "state"=w1314, "dev_type"=DEF_dev_type."devA (analyzer)", "dll_path"=w1313) -> ("error out"=w1310:errorcluster, "path out"=w1311:path)  [unwired: 2 in]
      }
      frame "release" {
        n684 = Dequeue Element(queue=w1324) -> ()  [unwired: 2 in, 4 out]
        n685 = flat-sequence {
          tunnel: w1323 -> [w1325]
          tunnel: w1319 -> [w1326]
          tunnel: [w1329] -> w1318
          tunnel: [w1328] -> w1317
          tunnel: [u32 0] -> w1316
          tunnel: [w1331] -> w1320
          tunnel: [w1332] -> w1321
          tunnel: [w1333] -> w1322
          tunnel: w1318 -> [w1333]
          tunnel: w1317 -> [w1332]
          tunnel: w1316 -> [w1331]
          frame #0 {
            n686 = call "SL2_AD_DLL_Phoibos_Shutdown.vi"("pHandle"=w1326, "dll path in"=w1325) -> ("error out"=w1328:errorcluster, "dll path out"=w1329:path)  [unwired: 4 in]
          }
          frame #1 {
            n687 = local write "phoib_con?"(FALSE ("phoib_con?")) -> ()
          }
        }
      }
      frame "close" {
        n688 = Release Queue(queue=w1338) -> ()  [unwired: 2 in, 3 out]
      }
      frame "suspend" {
        n689 = Dequeue Element(queue=w1342) -> ()  [unwired: 2 in, 4 out]
      }
      frame "init" {
        n690 = Dequeue Element(queue=w1348) -> ()  [unwired: 2 in, 4 out]
        n691 = flat-sequence {
          tunnel: [w1355] -> w1346
          tunnel: [w1351] -> w1345
          tunnel: [w1350] -> w1344
          tunnel: [w1363] -> w1347
          tunnel: w1346 -> [w1363]
          frame #0 {
            n692 = local write "phoib_con?"(FALSE ("phoib_con?")) -> ()
          }
          frame #1 {
            w1354 = DEF_dev_type."devA (analyzer)" ("dev_type")
            n693 = call "GetSL2AD_VI_dllPath.vi"() -> ("error"=w1358:errorcluster, "Path"=w1359:path)  [unwired: 9 in, 1 out]
            n694 = call "SL2_AD_DLL_List_Devices.vi"("error in"=w1358, "dev_type"=w1354, "dll path in"=w1359) -> ("error out"=w1352:errorcluster, "devices"=w1361:string[], "dll path out"=w1353:path)  [unwired: 2 in]
            n695 = Index Array(array=w1361) -> (element=w1360:string)  [unwired: 1 in]
            n696 = call "SL2_AD_DLL_Phoibos_Initialize.vi"("error in"=w1352, "analyzerId"=w1360, "dll_path"=w1353) -> ("error out"=w1356:errorcluster, "pHandle"=w1355:u32, "path out"=w1357:path)  [unwired: 2 in]
            n697 = call "SL2_AD_DLL_Phoibos_ListDeviceModes.vi"("dll path in"=w1357, "dev_type"=w1354, "pHandle"=w1355, "error in"=w1356) -> ("dll path out"=w1351:path, "error out"=w1350:errorcluster)  [unwired: 1 in, 2 out]
          }
          frame #2 {
            n698 = local write "phoib_con?"(TRUE ("phoib_con?")) -> ()
          }
        }
      }
    }
    "phoib_error" <- w1229
  }
